vi "OCV Histogram.vi"() -> ()   [LabVIEW 2019]
uses:
  OCVResults.ctl
  <vilib>/Analysis/baseanly.llb/Mean (DBL).vi
  <vilib>/Analysis/NI_AALBase.lvlib
  <vilib>/gmath/NI_Gmath.lvlib
panel:
  in  "Shorted at Pogo Pins":T1={"V ch0 Array"=[-4.644502656163076e-06, -5.008064093958253e-06, -5.142051723342297e-06, -4.750005660824572e-06, -4.652031142446432e-06, -5.209066755986695e-06, -5.091916834616591e-06, -4.630381027105227e-06, -5.21237404687769e-06, -5.620858205189846e-06, -5.343550677180362e-06, -6.185703766713982e-06, -5.671664561333461e-06, -5.927670894878171e-06, -5.546613668877613e-06, -6.364344983296889e-06, -6.520646681657183e-06, -6.284866762207373e-06, -6.533935582056949e-06, -6.4689426016067465e-06, -6.593996925988968e-06, -6.285432522003292e-06, -6.408103781833046e-06, -7.058105327323116e-06, -6.870211305723346e-06, -6.925936314908492e-06, -7.1087845232367935e-06, -6.979415887004172e-06, -7.113203152470592e-06, -6.8704523945523955e-06, -7.009159603790376e-06, -7.342517581426176e-06, -7.669098159443e-06, -7.489677328220809e-06, -7.132610877720342e-06, -7.304233870876275e-06, -7.66832379992834e-06, -7.715296105424593e-06, -7.986434127352774e-06, -7.898970931824006e-06], "V ch1 Array"=[4.7742232260821556e-06, 4.920022255268294e-06, 4.483256762256209e-06, 4.404065475875136e-06, 4.4716932731421325e-06, 4.548985062890386e-06, 4.522408472375412e-06, 4.095669599355476e-06, 3.999328189678911e-06, 3.6813476852782265e-06, 3.872005693197737e-06, 3.758508170269238e-06, 3.70571748427637e-06, 3.4759885510773306e-06, 2.9599721164895703e-06, 2.7610141257932504e-06, 2.8118433858193503e-06, 2.7104175464413036e-06, 2.565833035431353e-06, 2.185911565670746e-06, 2.685980675088301e-06, 2.6488195890091604e-06, 2.076266606944392e-06, 2.2698362478026414e-06, 1.5578322743180792e-06, 1.5376996626048395e-06, 1.150473677761539e-06, 1.8236979091692574e-06, 1.510963150770623e-06, 1.4855862808683257e-06, 1.4125163986427117e-06, 1.0735262618997076e-06, 9.45720576216451e-07, 4.7672136505507866e-07, 9.053063870402968e-07, 6.054055041162458e-07, 4.721349816794846e-07, 5.456028909058344e-07, 3.3431927350417376e-07, -1.5058882941009345e-07], "V ch2 Array"=[1.4134743604832099e-05, 1.3658244443019425e-05, 1.3479236357815262e-05, 1.367186906530213e-05, 1.2455842044663626e-05, 1.3434705047662445e-05, 1.3432391541088278e-05, 1.2888375409531819e-05, 1.2977936688443777e-05, 1.2674364164577651e-05, 1.2242971027474285e-05, 1.2123410935032508e-05, 1.1563631234108194e-05, 1.1923757910255661e-05, 1.1189143138664649e-05, 1.0898907804721548e-05, 1.0581785706128752e-05, 1.056110705533516e-05, 1.0471726258982195e-05, 1.0112137397062614e-05, 1.0207095545974621e-05, 1.0393895961777352e-05, 9.905291985333096e-06, 9.553343876750542e-06, 8.558186802328226e-06, 8.88351705449872e-06, 7.898230501439385e-06, 8.415417566964899e-06, 8.559435016019298e-06, 7.776376116877038e-06, 7.927651129172682e-06, 7.5739375202025605e-06, 7.10207278100178e-06, 6.5660504928688425e-06, 7.061106613490489e-06, 6.858259813662034e-06, 6.848030448614549e-06, 6.09752727757034e-06, 6.274361642967703e-06, 6.342704065028583e-06], "V ch3 Array"=[6.213352398330788e-06, 6.334228296782694e-06, 6.080028793939261e-06, 6.247654310029223e-06, 5.7595966055769634e-06, 5.814589345926128e-06, 5.6246681289139826e-06, 5.644165962745353e-06, 5.6293504739542166e-06, 5.352467720756411e-06, 5.130425551487793e-06, 5.1973648252728e-06, 5.044212335842026e-06, 4.8718454017924225e-06, 4.157122967118985e-06, 4.067943871712763e-06, 4.140736203520263e-06, 3.6541795943306613e-06, 4.0305384502788036e-06, 4.0890937751910164e-06, 3.7562699778786177e-06, 3.6969730552191906e-06, 3.508773289214503e-06, 3.4081260252248884e-06, 2.849755744581444e-06, 2.9121416252580047e-06, 2.743264262706753e-06, 2.425566322314393e-06, 2.3612672502798895e-06, 2.3528107196359356e-06, 2.284734780010105e-06, 2.0191213502578e-06, 1.7636078290436924e-06, 2.2789345039783042e-06, 1.9002135193771114e-06, 1.991552898527243e-06, 1.8062353830205049e-06, 1.382185125377262e-06, 1.10266330045512e-06, 1.2689722392645079e-06], "V ch4 Array"=[7.418128083831304e-06, 6.737017232964174e-06, 7.37695117366581e-06, 7.383316471897266e-06, 6.9171589884302516e-06, 6.824032641156624e-06, 7.123351361466038e-06, 6.907639604422655e-06, 6.77516452363689e-06, 6.995953660130747e-06, 6.47180172880639e-06, 6.431905767977081e-06, 6.870003361647515e-06, 6.6674721347179e-06, 6.65655896542764e-06, 5.8891322446061865e-06, 6.26132019363544e-06, 5.653457993699113e-06, 5.979464421600547e-06, 6.0940365547306505e-06, 5.726374609261477e-06, 5.609776313356894e-06, 5.925170773010799e-06, 5.980594209927675e-06, 5.615200324832046e-06, 5.423645487579083e-06, 4.863795777172752e-06, 5.24223894551309e-06, 4.7771857502833714e-06, 5.20649511681379e-06, 4.976881377243475e-06, 4.382659410631824e-06, 4.409179837473124e-06, 5.0132045585108375e-06, 4.846028587433284e-06, 5.007743407280303e-06, 5.115217349204208e-06, 4.756883872606744e-06, 4.378539859901796e-06, 4.191624122691694e-06], "Elapsed Time (ms)"=41178, "DMM Fault Array"=[FALSE, FALSE, FALSE, FALSE, FALSE, FALSE, FALSE, FALSE, FALSE, FALSE, FALSE, FALSE, FALSE, FALSE, FALSE, FALSE, FALSE, FALSE, FALSE, FALSE, FALSE, FALSE, FALSE, FALSE, FALSE, FALSE, FALSE, FALSE, FALSE, FALSE, FALSE, FALSE, FALSE, FALSE, FALSE, FALSE, FALSE, FALSE, FALSE, FALSE, FALSE, FALSE, FALSE, FALSE, FALSE, FALSE, FALSE, FALSE, FALSE, FALSE, FALSE, FALSE, FALSE, FALSE, FALSE, FALSE, FALSE, FALSE, FALSE, FALSE, FALSE, FALSE, FALSE, FALSE, FALSE, FALSE, FALSE, FALSE, FALSE, FALSE, FALSE, FALSE, FALSE, FALSE, FALSE, FALSE, FALSE, FALSE, FALSE, FALSE, FALSE, FALSE, FALSE, FALSE, FALSE, FALSE, FALSE, FALSE, FALSE, FALSE, FALSE, FALSE, FALSE, FALSE, FALSE, FALSE, FALSE, FALSE, FALSE, FALSE, FALSE, FALSE, FALSE, FALSE, FALSE, FALSE, FALSE, FALSE, FALSE, FALSE, FALSE, FALSE, FALSE, FALSE, FALSE, FALSE, FALSE, FALSE, FALSE, FALSE, FALSE, FALSE, FALSE, FALSE, FALSE, FALSE, FALSE, FALSE, FALSE, FALSE, FALSE, FALSE, FALSE, FALSE, FALSE, FALSE, FALSE, FALSE, FALSE, FALSE, FALSE, FALSE, FALSE, FALSE, FALSE, FALSE, FALSE, FALSE, FALSE, FALSE, FALSE, FALSE, FALSE, FALSE, FALSE, FALSE, FALSE, FALSE, FALSE, FALSE, FALSE, FALSE, FALSE, FALSE, FALSE, FALSE, FALSE, FALSE, FALSE, FALSE, FALSE, FALSE, FALSE, FALSE, FALSE, FALSE, FALSE, FALSE, FALSE, FALSE, FALSE, FALSE, FALSE, FALSE, FALSE, FALSE, FALSE, FALSE, FALSE, FALSE, FALSE, FALSE, FALSE, FALSE, FALSE, FALSE, FALSE, FALSE, FALSE, FALSE]}
  out "mean values of channels":dbl[](array[numeric])=[3.4860065278089722, 3.48375553663424, 3.4808778023254034, 3.484652928409848, 3.4829310355717924] format="%#_7p"
  in  "Aperture 200ms":T1={"V ch0 Array"=[3.486008136472735, 3.48600857919526, 3.486008593885945, 3.486008866783261, 3.48600839296004, 3.4860084310246897, 3.4860079537562934, 3.486008185287128, 3.486007910716225, 3.486008248243466, 3.486008226064088, 3.4860074977647457, 3.4860073987599094, 3.4860073866023904, 3.486006180409399, 3.486007074730973, 3.486007704925445, 3.4860074052013497, 3.4860071909298775, 3.486007294352636, 3.4860070893197057, 3.486006585724478, 3.4860062950330795, 3.486005770351729, 3.486006470228577, 3.486006294219978, 3.486006261625677, 3.486005971624855, 3.4860053268849924, 3.486005293813216, 3.4860057372410087, 3.4860055538519807, 3.486004986165897, 3.486005215637336, 3.4860050104743285, 3.4860054747400397, 3.486005352423458, 3.486005243822349, 3.4860053543618483, 3.4860050193699643], "V ch1 Array"=[3.483761574282832, 3.4837611271000504, 3.483761800210414, 3.4837619249854033, 3.4837611548851593, 3.483760899396786, 3.483761030316352, 3.4837614126693177, 3.483761111670994, 3.483761223907113, 3.4837605553855715, 3.483760811426642, 3.483760756142808, 3.483760849802524, 3.48376001298478, 3.4837605620529932, 3.483760624523579, 3.4837598644530314, 3.4837598021350367, 3.483759678841745, 3.483759236759767, 3.483759830079179, 3.4837586449222844, 3.4837592160716793, 3.4837591729619493, 3.4837584791863603, 3.4837585600417578, 3.483758759299516, 3.483758443826462, 3.4837582905594657, 3.483758319275863, 3.4837578525324924, 3.483757492097309, 3.483758508843088, 3.483758252435504, 3.4837583290172742, 3.4837582653066366, 3.4837580432257322, 3.4837579872411233, 3.4837572297984027], "V ch2 Array"=[3.480887331125, 3.4808873642804303, 3.4808872284950985, 3.4808870880116816, 3.480886718645805, 3.480886569722079, 3.480886668360947, 3.480887124574677, 3.4808868556225554, 3.4808863352702843, 3.480886374563708, 3.4808863195405926, 3.480885492039432, 3.480885499125927, 3.4808853435833824, 3.480885304255472, 3.4808854048927067, 3.480885548024527, 3.4808846074916104, 3.480884933260716, 3.480884045102653, 3.4808848759996445, 3.4808834564381117, 3.480884092168976, 3.4808840639635292, 3.4808839119975015, 3.480884117918731, 3.4808838222854104, 3.4808837132230104, 3.480882970525138, 3.4808832280724213, 3.480882799469968, 3.4808825004595314, 3.4808829485765864, 3.4808825054329224, 3.480882618811386, 3.480882555023867, 3.4808814816354365, 3.4808821449010603, 3.480881613246818], "V ch3 Array"=[3.4846494420325933, 3.4846499531928408, 3.484649881478528, 3.484649477663704, 3.484649028003101, 3.4846491662272117, 3.484648764064297, 3.484649038455092, 3.4846488791274033, 3.4846493802112795, 3.484648500366631, 3.4846488541657643, 3.484647926389134, 3.484647926012707, 3.4846477409134877, 3.4846480348803968, 3.4846481902030244, 3.4846476677611595, 3.484647180925758, 3.4846471596264443, 3.48464679726762, 3.484647693286154, 3.484646021250072, 3.4846464856341806, 3.48464646608778, 3.4846465629811068, 3.4846461202335623, 3.484646282076445, 3.484645610465135, 3.4846448549897504, 3.484645234223203, 3.484644743913154, 3.4846449104812334, 3.484645286668683, 3.4846446745957183, 3.4846443026433325, 3.484644591867837, 3.484643852000993, 3.4846443663887183, 3.4846437781492234], "V ch4 Array"=[3.4829266330342312, 3.482927618195819, 3.4829267375359523, 3.482926673878544, 3.482926361108386, 3.482926051177458, 3.4829261918098164, 3.482926643011778, 3.4829263973622697, 3.4829267486003386, 3.482926239361367, 3.482926009047662, 3.4829255763196625, 3.4829252649644946, 3.482926010999456, 3.4829256561545856, 3.482925616603878, 3.482925430299697, 3.482925384824906, 3.482925111093104, 3.4829243773568472, 3.4829245855818627, 3.4829236684214164, 3.4829243150207865, 3.48292388842584, 3.482924459144899, 3.4829244509598785, 3.4829235506462766, 3.4829238640017737, 3.4829231152951126, 3.4829231533373095, 3.4829234989073856, 3.482923429513632, 3.482923569887466, 3.4829233778303514, 3.48292294148491, 3.4829225870708402, 3.482922885194255, 3.48292277091393, 3.482922191039904], "Elapsed Time (ms)"=41179, "DMM Fault Array"=[FALSE, FALSE, FALSE, FALSE, FALSE, FALSE, FALSE, FALSE, FALSE, FALSE, FALSE, FALSE, FALSE, FALSE, FALSE, FALSE, FALSE, FALSE, FALSE, FALSE, FALSE, FALSE, FALSE, FALSE, FALSE, FALSE, FALSE, FALSE, FALSE, FALSE, FALSE, FALSE, FALSE, FALSE, FALSE, FALSE, FALSE, FALSE, FALSE, FALSE, FALSE, FALSE, FALSE, FALSE, FALSE, FALSE, FALSE, FALSE, FALSE, FALSE, FALSE, FALSE, FALSE, FALSE, FALSE, FALSE, FALSE, FALSE, FALSE, FALSE, FALSE, FALSE, FALSE, FALSE, FALSE, FALSE, FALSE, FALSE, FALSE, FALSE, FALSE, FALSE, FALSE, FALSE, FALSE, FALSE, FALSE, FALSE, FALSE, FALSE, FALSE, FALSE, FALSE, FALSE, FALSE, FALSE, FALSE, FALSE, FALSE, FALSE, FALSE, FALSE, FALSE, FALSE, FALSE, FALSE, FALSE, FALSE, FALSE, FALSE, FALSE, FALSE, FALSE, FALSE, FALSE, FALSE, FALSE, FALSE, FALSE, FALSE, FALSE, FALSE, FALSE, FALSE, FALSE, FALSE, FALSE, FALSE, FALSE, FALSE, FALSE, FALSE, FALSE, FALSE, FALSE, FALSE, FALSE, FALSE, FALSE, FALSE, FALSE, FALSE, FALSE, FALSE, FALSE, FALSE, FALSE, FALSE, FALSE, FALSE, FALSE, FALSE, FALSE, FALSE, FALSE, FALSE, FALSE, FALSE, FALSE, FALSE, FALSE, FALSE, FALSE, FALSE, FALSE, FALSE, FALSE, FALSE, FALSE, FALSE, FALSE, FALSE, FALSE, FALSE, FALSE, FALSE, FALSE, FALSE, FALSE, FALSE, FALSE, FALSE, FALSE, FALSE, FALSE, FALSE, FALSE, FALSE, FALSE, FALSE, FALSE, FALSE, FALSE, FALSE, FALSE, FALSE, FALSE, FALSE, FALSE, FALSE, FALSE, FALSE, FALSE, FALSE, FALSE, FALSE, FALSE, FALSE, FALSE, FALSE]}
  in  "Aperture 100ms":T1={"V ch0 Array"=[3.486009342585924, 3.4860105791739295, 3.486009931293131, 3.4860104287389, 3.4860092107388985, 3.486010141865981, 3.4860099876219555, 3.4860099847912083, 3.4860105815524287, 3.4860097585412158, 3.486009884787763, 3.4860103699490104, 3.4860101319846923, 3.4860100232587925, 3.4860097575418165, 3.4860098656116585, 3.4860099281665464, 3.4860101703729627, 3.4860095171681698, 3.486009274858784, 3.486008835388769, 3.4860101964727264, 3.4860099208454622, 3.486009396754712, 3.486009765859615, 3.4860100085572148, 3.486009761006136, 3.4860093507563175, 3.486010114650017, 3.486010095359039, 3.486009239422696, 3.486009747196399, 3.4860095662543613, 3.486009897920948, 3.4860090987744554, 3.4860091306648, 3.4860088161589653, 3.4860087248708242, 3.486008795417955, 3.4860089917588786], "V ch1 Array"=[3.4837624269768077, 3.48376228114691, 3.4837624931669393, 3.483761690503522, 3.483762155112424, 3.4837623742938635, 3.483762530621196, 3.4837625073929708, 3.4837629531752388, 3.4837628311532667, 3.4837623445473884, 3.4837624893774435, 3.4837624783754726, 3.4837629314944056, 3.4837620420976028, 3.4837623355175706, 3.4837620224590617, 3.4837628211868528, 3.4837625542351085, 3.4837617678834287, 3.4837613820224265, 3.4837629202530915, 3.483762550398443, 3.483762098662157, 3.483762194447779, 3.483762525958178, 3.4837624272950842, 3.4837620308215613, 3.4837620769856987, 3.483762428084855, 3.4837614921239366, 3.4837618093626643, 3.483761940909492, 3.483762461616833, 3.483761691185677, 3.4837617745493117, 3.483761713223301, 3.4837616040814634, 3.4837614420599667, 3.48376097030803], "V ch2 Array"=[3.4808881795721174, 3.4808883313716246, 3.480888898340563, 3.480888295742587, 3.480888608550977, 3.4808887791773486, 3.4808884610442696, 3.480888665380878, 3.4808884002018616, 3.4808887742205608, 3.480887630055783, 3.4808880675947815, 3.4808884701480265, 3.4808883902919048, 3.4808881624179406, 3.4808878492628614, 3.480888261000973, 3.4808883629946665, 3.4808881818180226, 3.4808876522799888, 3.480887461292375, 3.480888607451478, 3.480887839077484, 3.4808872769077657, 3.4808874503677765, 3.4808875084242965, 3.4808873046245945, 3.4808874834171952, 3.480886785383865, 3.480886872329251, 3.4808875891233906, 3.480887116764498, 3.480886791395762, 3.480887286883312, 3.4808869352248015, 3.4808867541286497, 3.4808863857441597, 3.480886392902343, 3.480886055482132, 3.480885490000428], "V ch3 Array"=[3.484651699388893, 3.484651545846978, 3.4846512315009237, 3.4846512380454784, 3.4846516053658094, 3.4846518730555442, 3.484651375621465, 3.4846524671533308, 3.484651872127177, 3.484651836357751, 3.4846512940631733, 3.484651339393445, 3.484651943755441, 3.484651992458054, 3.484650533966351, 3.484650906778825, 3.4846514868400833, 3.4846515569158076, 3.4846513629276004, 3.4846508460654917, 3.484650626430101, 3.4846512615447227, 3.4846506421425434, 3.484651362249249, 3.4846503023743085, 3.4846507344492568, 3.484650635547321, 3.4846504986168716, 3.484650507900654, 3.484650249934964, 3.484650813855195, 3.484649807825047, 3.484649765228285, 3.48465038699218, 3.484649863980596, 3.484649023843705, 3.4846489818429665, 3.484649383129509, 3.484649201493699, 3.4846489918759493], "V ch4 Array"=[3.482927735803894, 3.482927340280007, 3.482927450118009, 3.482927667247653, 3.482927828334824, 3.4829274360243563, 3.482928060851357, 3.4829282380460005, 3.482927707338127, 3.482927638010684, 3.48292776532699, 3.4829276207246203, 3.482928248308542, 3.4829279098062047, 3.4829276721732416, 3.4829277669695853, 3.4829282785856024, 3.4829278902480967, 3.482927734684043, 3.482927119973658, 3.482927618691812, 3.482927625774665, 3.4829269275383856, 3.4829274148488474, 3.4829274061226, 3.4829269572792154, 3.4829273071837483, 3.482928083458411, 3.482928213245571, 3.4829277993020136, 3.4829274353081385, 3.4829265960951377, 3.4829273450195637, 3.4829272886160374, 3.4829269443181414, 3.482926203898658, 3.4829261490935757, 3.4829262414280016, 3.4829262680441184, 3.482925750053477], "Elapsed Time (ms)"=21179, "DMM Fault Array"=[FALSE, FALSE, FALSE, FALSE, FALSE, FALSE, FALSE, FALSE, FALSE, FALSE, FALSE, FALSE, FALSE, FALSE, FALSE, FALSE, FALSE, FALSE, FALSE, FALSE, FALSE, FALSE, FALSE, FALSE, FALSE, FALSE, FALSE, FALSE, FALSE, FALSE, FALSE, FALSE, FALSE, FALSE, FALSE, FALSE, FALSE, FALSE, FALSE, FALSE, FALSE, FALSE, FALSE, FALSE, FALSE, FALSE, FALSE, FALSE, FALSE, FALSE, FALSE, FALSE, FALSE, FALSE, FALSE, FALSE, FALSE, FALSE, FALSE, FALSE, FALSE, FALSE, FALSE, FALSE, FALSE, FALSE, FALSE, FALSE, FALSE, FALSE, FALSE, FALSE, FALSE, FALSE, FALSE, FALSE, FALSE, FALSE, FALSE, FALSE, FALSE, FALSE, FALSE, FALSE, FALSE, FALSE, FALSE, FALSE, FALSE, FALSE, FALSE, FALSE, FALSE, FALSE, FALSE, FALSE, FALSE, FALSE, FALSE, FALSE, FALSE, FALSE, FALSE, FALSE, FALSE, FALSE, FALSE, FALSE, FALSE, FALSE, FALSE, FALSE, FALSE, FALSE, FALSE, FALSE, FALSE, FALSE, FALSE, FALSE, FALSE, FALSE, FALSE, FALSE, FALSE, FALSE, FALSE, FALSE, FALSE, FALSE, FALSE, FALSE, FALSE, FALSE, FALSE, FALSE, FALSE, FALSE, FALSE, FALSE, FALSE, FALSE, FALSE, FALSE, FALSE, FALSE, FALSE, FALSE, FALSE, FALSE, FALSE, FALSE, FALSE, FALSE, FALSE, FALSE, FALSE, FALSE, FALSE, FALSE, FALSE, FALSE, FALSE, FALSE, FALSE, FALSE, FALSE, FALSE, FALSE, FALSE, FALSE, FALSE, FALSE, FALSE, FALSE, FALSE, FALSE, FALSE, FALSE, FALSE, FALSE, FALSE, FALSE, FALSE, FALSE, FALSE, FALSE, FALSE, FALSE, FALSE, FALSE, FALSE, FALSE, FALSE, FALSE, FALSE, FALSE, FALSE, FALSE, FALSE]}
  in  "Aperture 83.333ms":T1={"V ch0 Array"=[3.486011308516991, 3.486012239712371, 3.4860117488002986, 3.4860117846643788, 3.4860112460509, 3.4860122062360275, 3.486011836169301, 3.486012369801971, 3.4860122187882556, 3.486012566602132, 3.4860122523310664, 3.4860122171529238, 3.4860121108134354, 3.4860123157743494, 3.4860122873127923, 3.4860124760718674, 3.486012337141422, 3.4860116684592, 3.4860121407169955, 3.4860121021406, 3.4860123592450254, 3.486012151457661, 3.486012121814877, 3.486012067279236, 3.4860123631776054, 3.4860121056043045, 3.4860114488809137, 3.486011754799218, 3.4860106856009794, 3.4860112875473717, 3.486011703795938, 3.4860120408526933, 3.4860107437568857, 3.48601088290282, 3.4860113654835745, 3.486011077482956, 3.486011198731769, 3.4860110498434973, 3.4860110418920347, 3.4860114222959866], "V ch1 Array"=[3.48376144514735, 3.483762834467521, 3.4837631670672375, 3.4837623545770247, 3.483762107595157, 3.4837626511367517, 3.483762686272187, 3.483763061857131, 3.483762799687585, 3.483763256237141, 3.4837627216036235, 3.4837630898972405, 3.4837625437622455, 3.483763470688663, 3.483763332566706, 3.4837632413297466, 3.4837632297716534, 3.483763046847993, 3.483762554574395, 3.4837626769665397, 3.483763593758579, 3.4837636694535936, 3.4837630032740696, 3.4837637224866063, 3.4837629548968807, 3.4837628958155715, 3.4837626640538226, 3.4837626122337526, 3.483762711500467, 3.483762055280072, 3.483762819116541, 3.4837627515538023, 3.483761992186221, 3.4837623338946315, 3.4837620187762153, 3.483761909221837, 3.483762264846845, 3.4837623892072913, 3.4837624615777685, 3.483762348335557], "V ch2 Array"=[3.480888708513571, 3.4808899222268774, 3.4808891805476914, 3.480890012447383, 3.4808892224486154, 3.4808893541433874, 3.4808892866436536, 3.480890020112137, 3.4808897263400347, 3.480889783586903, 3.480889935849121, 3.4808896507279634, 3.480889351773294, 3.480890064216353, 3.4808901385444586, 3.4808896580000983, 3.480889498764669, 3.4808898293598274, 3.4808895506765243, 3.480889693145708, 3.480889162389052, 3.4808896927476467, 3.4808892966308354, 3.4808899571134586, 3.480889465662438, 3.4808889111399703, 3.480888409068941, 3.480888525715946, 3.4808890429173713, 3.4808889264302345, 3.4808885737492994, 3.480888487697757, 3.480888024775162, 3.4808879516614852, 3.4808876036613943, 3.4808880185797495, 3.4808879533956265, 3.4808879726788993, 3.4808881120797213, 3.480887678005953], "V ch3 Array"=[3.4846535014569993, 3.4846541760292356, 3.484653522898726, 3.4846537234499997, 3.484654274868219, 3.4846541533184623, 3.4846538790205623, 3.484653703267222, 3.4846537737054746, 3.484654159822945, 3.484654165902905, 3.484654192635321, 3.484654175425727, 3.4846535327376635, 3.484653580198149, 3.484654506816064, 3.4846534264712856, 3.484653785252615, 3.484653990393246, 3.4846533736484147, 3.4846532689913223, 3.484653468831708, 3.4846538432365963, 3.4846537804540145, 3.4846535567722334, 3.4846528159762866, 3.4846519071808677, 3.4846523265662555, 3.484652590816005, 3.484651964351458, 3.4846524738855367, 3.4846523590459872, 3.484652375375891, 3.484652087227577, 3.484651774761584, 3.484651925046, 3.4846519185425966, 3.4846519450610187, 3.4846520067304745, 3.4846515142009595], "V ch4 Array"=[3.4829264000035693, 3.4829270474083764, 3.4829273700349654, 3.48292728310475, 3.482927554955438, 3.4829280842549744, 3.482928116817796, 3.4829269335611985, 3.4829284615526284, 3.4829276929963067, 3.482928105095857, 3.4829276890211416, 3.482927228135068, 3.482927749550447, 3.4829278369724954, 3.4829277993952084, 3.482928003490174, 3.4829275404308224, 3.48292756348699, 3.482927639736477, 3.482926867361093, 3.4829272666686393, 3.482927349826675, 3.482927777135856, 3.482926506905905, 3.482926708523178, 3.482927039514058, 3.482926967607869, 3.482926263410761, 3.482926437644337, 3.4829274705024393, 3.482926618936467, 3.482926341189578, 3.48292661596785, 3.4829265616882217, 3.4829265081437066, 3.4829261104994833, 3.4829263487877005, 3.4829268727396743, 3.4829262442480986], "Elapsed Time (ms)"=17840, "DMM Fault Array"=[FALSE, FALSE, FALSE, FALSE, FALSE, FALSE, FALSE, FALSE, FALSE, FALSE, FALSE, FALSE, FALSE, FALSE, FALSE, FALSE, FALSE, FALSE, FALSE, FALSE, FALSE, FALSE, FALSE, FALSE, FALSE, FALSE, FALSE, FALSE, FALSE, FALSE, FALSE, FALSE, FALSE, FALSE, FALSE, FALSE, FALSE, FALSE, FALSE, FALSE, FALSE, FALSE, FALSE, FALSE, FALSE, FALSE, FALSE, FALSE, FALSE, FALSE, FALSE, FALSE, FALSE, FALSE, FALSE, FALSE, FALSE, FALSE, FALSE, FALSE, FALSE, FALSE, FALSE, FALSE, FALSE, FALSE, FALSE, FALSE, FALSE, FALSE, FALSE, FALSE, FALSE, FALSE, FALSE, FALSE, FALSE, FALSE, FALSE, FALSE, FALSE, FALSE, FALSE, FALSE, FALSE, FALSE, FALSE, FALSE, FALSE, FALSE, FALSE, FALSE, FALSE, FALSE, FALSE, FALSE, FALSE, FALSE, FALSE, FALSE, FALSE, FALSE, FALSE, FALSE, FALSE, FALSE, FALSE, FALSE, FALSE, FALSE, FALSE, FALSE, FALSE, FALSE, FALSE, FALSE, FALSE, FALSE, FALSE, FALSE, FALSE, FALSE, FALSE, FALSE, FALSE, FALSE, FALSE, FALSE, FALSE, FALSE, FALSE, FALSE, FALSE, FALSE, FALSE, FALSE, FALSE, FALSE, FALSE, FALSE, FALSE, FALSE, FALSE, FALSE, FALSE, FALSE, FALSE, FALSE, FALSE, FALSE, FALSE, FALSE, FALSE, FALSE, FALSE, FALSE, FALSE, FALSE, FALSE, FALSE, FALSE, FALSE, FALSE, FALSE, FALSE, FALSE, FALSE, FALSE, FALSE, FALSE, FALSE, FALSE, FALSE, FALSE, FALSE, FALSE, FALSE, FALSE, FALSE, FALSE, FALSE, FALSE, FALSE, FALSE, FALSE, FALSE, FALSE, FALSE, FALSE, FALSE, FALSE, FALSE, FALSE, FALSE, FALSE, FALSE, FALSE, FALSE, FALSE, FALSE]}
  in  "Aperture 66.666ms":T1={"V ch0 Array"=[3.4860087998577005, 3.4860095881357007, 3.4860101243172754, 3.4860101144901403, 3.486009888487567, 3.4860095771678257, 3.486009669258281, 3.4860094591080513, 3.4860103646585396, 3.4860097369646823, 3.4860096987264826, 3.486009571351648, 3.4860098771934167, 3.4860097835806916, 3.486009561905741, 3.486010032506046, 3.4860089841340414, 3.4860092949017023, 3.4860102057709037, 3.4860095439580023, 3.486010152423206, 3.4860106769541708, 3.486010233961671, 3.4860094919269367, 3.4860097824232867, 3.4860095692285054, 3.486009586955168, 3.486009895817203, 3.486010327033842, 3.486009759381219, 3.4860098017300087, 3.4860101603499363, 3.4860098840038014, 3.4860099658133556, 3.486009908145774, 3.486009609018681, 3.4860096586646816, 3.486009804783706, 3.4860093085592134, 3.486009478902439], "V ch1 Array"=[3.483760919705666, 3.483761869245746, 3.483761959360454, 3.4837610510443393, 3.4837611770683603, 3.4837613541505483, 3.483761535168446, 3.4837615945078113, 3.483762097514668, 3.4837613706486406, 3.483761473980138, 3.483761884265854, 3.4837617247467976, 3.4837617012079223, 3.483760834123308, 3.483761090501802, 3.48376059513931, 3.4837613052709315, 3.483762005734639, 3.4837610896972415, 3.4837617908589684, 3.4837615663936834, 3.483761747238985, 3.4837616692609985, 3.483761646197544, 3.483761294896974, 3.4837604944369978, 3.483761837306543, 3.4837615877681896, 3.4837618075102377, 3.4837615882889503, 3.483761703673241, 3.483761248077784, 3.483761700151896, 3.4837612726209124, 3.483760588068086, 3.4837613416844158, 3.4837609694613487, 3.483760924435762, 3.4837608925182137], "V ch2 Array"=[3.4808863773772543, 3.480886669418454, 3.4808873886157263, 3.480886413588629, 3.4808873618899736, 3.4808873437807266, 3.480886755177445, 3.4808869453382223, 3.480887464165299, 3.480886900782393, 3.4808870436569843, 3.4808874679648922, 3.4808870994368517, 3.4808865690442543, 3.480886784455878, 3.4808868210363446, 3.4808859487488313, 3.4808868680223597, 3.480886776757931, 3.480886801707026, 3.480887196454042, 3.480887405892581, 3.4808876132499544, 3.480886555301745, 3.480886529704909, 3.480886739877629, 3.4808865320412967, 3.480887301554799, 3.480886582542384, 3.4808868800235953, 3.480886739982213, 3.4808867859782278, 3.4808864774264436, 3.480886305721363, 3.4808861528966646, 3.4808867325743194, 3.4808864343840265, 3.480886312203627, 3.480886584938389, 3.48088646297481], "V ch3 Array"=[3.484650807229959, 3.484651774283296, 3.4846519516933347, 3.4846516319475054, 3.484652063235418, 3.484652071854816, 3.4846516202986617, 3.4846517014537373, 3.4846523194092835, 3.4846521211999524, 3.484651702162199, 3.4846519295670677, 3.4846517340825005, 3.4846513680635502, 3.4846512057138934, 3.4846515287948328, 3.4846519286333084, 3.484651188287481, 3.484651349773111, 3.484651995793708, 3.4846520150992184, 3.4846522758834984, 3.4846518137849802, 3.484651297913903, 3.4846510243965803, 3.484651358305008, 3.484651452402426, 3.4846524632395934, 3.484651705527652, 3.484651694168373, 3.4846516821692313, 3.4846512991773837, 3.4846514629860112, 3.484650672181916, 3.4846509088214157, 3.484650732648704, 3.484650894748678, 3.4846505911642187, 3.484651294143712, 3.4846510357548985], "V ch4 Array"=[3.4829272996810947, 3.4829272782624443, 3.4829275139775517, 3.4829269004471395, 3.4829275408550995, 3.4829277689113125, 3.4829271335226237, 3.4829276730931262, 3.4829268209667936, 3.482927367613094, 3.482927607066623, 3.4829268691426827, 3.4829268903447055, 3.4829273896280197, 3.482927105499838, 3.4829262932216025, 3.482927081371735, 3.4829266027300334, 3.48292673298539, 3.482927489707926, 3.48292727137664, 3.4829276427095914, 3.4829278822666185, 3.482926515712328, 3.482926621734275, 3.482927051972468, 3.48292694912251, 3.4829277226679234, 3.482927064940792, 3.4829270499583376, 3.482927283643157, 3.482927446903043, 3.482927333199049, 3.482926437014769, 3.48292713227865, 3.482926646534637, 3.482926836756891, 3.482926598365688, 3.482926850846762, 3.4829269468668755], "Elapsed Time (ms)"=14513, "DMM Fault Array"=[FALSE, FALSE, FALSE, FALSE, FALSE, FALSE, FALSE, FALSE, FALSE, FALSE, FALSE, FALSE, FALSE, FALSE, FALSE, FALSE, FALSE, FALSE, FALSE, FALSE, FALSE, FALSE, FALSE, FALSE, FALSE, FALSE, FALSE, FALSE, FALSE, FALSE, FALSE, FALSE, FALSE, FALSE, FALSE, FALSE, FALSE, FALSE, FALSE, FALSE, FALSE, FALSE, FALSE, FALSE, FALSE, FALSE, FALSE, FALSE, FALSE, FALSE, FALSE, FALSE, FALSE, FALSE, FALSE, FALSE, FALSE, FALSE, FALSE, FALSE, FALSE, FALSE, FALSE, FALSE, FALSE, FALSE, FALSE, FALSE, FALSE, FALSE, FALSE, FALSE, FALSE, FALSE, FALSE, FALSE, FALSE, FALSE, FALSE, FALSE, FALSE, FALSE, FALSE, FALSE, FALSE, FALSE, FALSE, FALSE, FALSE, FALSE, FALSE, FALSE, FALSE, FALSE, FALSE, FALSE, FALSE, FALSE, FALSE, FALSE, FALSE, FALSE, FALSE, FALSE, FALSE, FALSE, FALSE, FALSE, FALSE, FALSE, FALSE, FALSE, FALSE, FALSE, FALSE, FALSE, FALSE, FALSE, FALSE, FALSE, FALSE, FALSE, FALSE, FALSE, FALSE, FALSE, FALSE, FALSE, FALSE, FALSE, FALSE, FALSE, FALSE, FALSE, FALSE, FALSE, FALSE, FALSE, FALSE, FALSE, FALSE, FALSE, FALSE, FALSE, FALSE, FALSE, FALSE, FALSE, FALSE, FALSE, FALSE, FALSE, FALSE, FALSE, FALSE, FALSE, FALSE, FALSE, FALSE, FALSE, FALSE, FALSE, FALSE, FALSE, FALSE, FALSE, FALSE, FALSE, FALSE, FALSE, FALSE, FALSE, FALSE, FALSE, FALSE, FALSE, FALSE, FALSE, FALSE, FALSE, FALSE, FALSE, FALSE, FALSE, FALSE, FALSE, FALSE, FALSE, FALSE, FALSE, FALSE, FALSE, FALSE, FALSE, FALSE, FALSE, FALSE, FALSE, FALSE, FALSE]}
  in  "Aperture 50ms":T1={"V ch0 Array"=[3.4860100287152176, 3.4860105188849553, 3.4860106708159453, 3.4860094634778664, 3.4860099118737806, 3.486010523724517, 3.4860099052381313, 3.4860102303967886, 3.4860101301121498, 3.486010292651811, 3.486010199771339, 3.4860106853911876, 3.4860109895623905, 3.4860107133588483, 3.486010447394096, 3.4860106566610725, 3.486010997892429, 3.4860101234952126, 3.48600996479348, 3.486010103181317, 3.4860105876357554, 3.48601023084213, 3.486009867094396, 3.4860098108988984, 3.4860092398388813, 3.486009725324624, 3.4860096603576003, 3.486008896488685, 3.4860092704556815, 3.4860095697732945, 3.486008558194004, 3.4860089610080696, 3.486008673120214, 3.4860087699924494, 3.4860092785317387, 3.486009367161149, 3.486009226546915, 3.4860096822694366, 3.4860096977392105, 3.4860099169280505], "V ch1 Array"=[3.4837622547034077, 3.4837615815666485, 3.483762529014476, 3.4837621681655278, 3.483762188707288, 3.4837618633463263, 3.483763227201614, 3.4837621427685534, 3.483762683392615, 3.4837623289394593, 3.4837627534166558, 3.48376346772014, 3.4837636251775055, 3.483762457405858, 3.4837634794729304, 3.483762977481437, 3.4837629345679324, 3.4837631030207246, 3.4837629456461694, 3.4837628484726055, 3.483761997597191, 3.4837625049740137, 3.483762216727805, 3.4837620043126956, 3.48376213159136, 3.483762096545265, 3.4837617435558927, 3.4837615058818554, 3.4837615885265003, 3.4837616255565362, 3.4837616788541252, 3.4837613812367385, 3.4837609512517314, 3.4837611696355744, 3.483761983589698, 3.483761966858258, 3.4837613659045283, 3.4837618682766567, 3.483761915919694, 3.4837619313026145], "V ch2 Array"=[3.4808869609246615, 3.480887261550433, 3.4808881245642356, 3.480887435501162, 3.4808866862045176, 3.480887868244338, 3.4808878821670226, 3.4808874703312456, 3.4808879690318433, 3.480888364513961, 3.480888033583846, 3.4808881142078136, 3.4808884304361305, 3.4808877278394137, 3.480888662188628, 3.480888094184551, 3.480887905268431, 3.480888371276923, 3.4808875432440796, 3.4808870941774988, 3.480887088434577, 3.480886791269301, 3.4808872805992475, 3.48088653865037, 3.4808866413425985, 3.4808865319189217, 3.48088656482604, 3.480886159814531, 3.4808860148618375, 3.480886538568749, 3.4808863033367845, 3.4808863711956852, 3.480886349091009, 3.480886181851329, 3.480886257965578, 3.4808862479847065, 3.4808864937119854, 3.480885765574369, 3.4808864743103074, 3.480887148388446], "V ch3 Array"=[3.4846509510160764, 3.4846510772479133, 3.4846514563068767, 3.4846511988461897, 3.4846505946638815, 3.4846512096738143, 3.4846517813774347, 3.4846511706468046, 3.4846511446643524, 3.4846514268988478, 3.4846516574479858, 3.4846511067785237, 3.4846520394102742, 3.484651878669274, 3.4846515793422235, 3.484651904943696, 3.4846511309148287, 3.4846514308431367, 3.4846516282787454, 3.484650023138923, 3.484651163887891, 3.484650193990817, 3.4846513598563225, 3.4846500346856906, 3.4846499656426575, 3.4846498234359946, 3.4846503795494663, 3.4846493936957663, 3.4846497630741227, 3.4846502843060607, 3.484649841027079, 3.4846493597248243, 3.484649892599996, 3.4846501778195464, 3.484650363201697, 3.484650494803555, 3.4846496243922878, 3.48464972852744, 3.4846500119053396, 3.484650533730012], "V ch4 Array"=[3.4829269850420745, 3.482927590238761, 3.482926653853842, 3.4829272143652914, 3.482927514085087, 3.482926705112038, 3.4829271862570357, 3.482926691178922, 3.482927613190633, 3.4829280914145424, 3.4829273547258395, 3.4829278085809356, 3.4829273448330196, 3.4829267716041663, 3.4829274831376797, 3.4829276839601047, 3.48292753499368, 3.48292751625691, 3.482926970155153, 3.482927468403634, 3.482927606619747, 3.482926889628744, 3.482927135801245, 3.4829262477892695, 3.4829270214994756, 3.4829260292107223, 3.4829260559211996, 3.482926067329125, 3.482926268835784, 3.482926248827354, 3.4829258919295123, 3.4829255437612, 3.482925544229328, 3.482925454846341, 3.4829265604884223, 3.4829256645431097, 3.482925571973606, 3.4829265171301365, 3.4829258623487998, 3.4829263404476105], "Elapsed Time (ms)"=11163, "DMM Fault Array"=[FALSE, FALSE, FALSE, FALSE, FALSE, FALSE, FALSE, FALSE, FALSE, FALSE, FALSE, FALSE, FALSE, FALSE, FALSE, FALSE, FALSE, FALSE, FALSE, FALSE, FALSE, FALSE, FALSE, FALSE, FALSE, FALSE, FALSE, FALSE, FALSE, FALSE, FALSE, FALSE, FALSE, FALSE, FALSE, FALSE, FALSE, FALSE, FALSE, FALSE, FALSE, FALSE, FALSE, FALSE, FALSE, FALSE, FALSE, FALSE, FALSE, FALSE, FALSE, FALSE, FALSE, FALSE, FALSE, FALSE, FALSE, FALSE, FALSE, FALSE, FALSE, FALSE, FALSE, FALSE, FALSE, FALSE, FALSE, FALSE, FALSE, FALSE, FALSE, FALSE, FALSE, FALSE, FALSE, FALSE, FALSE, FALSE, FALSE, FALSE, FALSE, FALSE, FALSE, FALSE, FALSE, FALSE, FALSE, FALSE, FALSE, FALSE, FALSE, FALSE, FALSE, FALSE, FALSE, FALSE, FALSE, FALSE, FALSE, FALSE, FALSE, FALSE, FALSE, FALSE, FALSE, FALSE, FALSE, FALSE, FALSE, FALSE, FALSE, FALSE, FALSE, FALSE, FALSE, FALSE, FALSE, FALSE, FALSE, FALSE, FALSE, FALSE, FALSE, FALSE, FALSE, FALSE, FALSE, FALSE, FALSE, FALSE, FALSE, FALSE, FALSE, FALSE, FALSE, FALSE, FALSE, FALSE, FALSE, FALSE, FALSE, FALSE, FALSE, FALSE, FALSE, FALSE, FALSE, FALSE, FALSE, FALSE, FALSE, FALSE, FALSE, FALSE, FALSE, FALSE, FALSE, FALSE, FALSE, FALSE, FALSE, FALSE, FALSE, FALSE, FALSE, FALSE, FALSE, FALSE, FALSE, FALSE, FALSE, FALSE, FALSE, FALSE, FALSE, FALSE, FALSE, FALSE, FALSE, FALSE, FALSE, FALSE, FALSE, FALSE, FALSE, FALSE, FALSE, FALSE, FALSE, FALSE, FALSE, FALSE, FALSE, FALSE, FALSE, FALSE, FALSE, FALSE, FALSE, FALSE]}
  in  "Aperture 33.333ms":T1={"V ch0 Array"=[3.486008824721795, 3.4860102954706935, 3.4860102805490536, 3.4860104842509556, 3.486010439216268, 3.4860097506123746, 3.4860094118729426, 3.4860095021603867, 3.486009978947523, 3.4860098527233068, 3.4860104496716957, 3.4860103895692003, 3.486010367848577, 3.48601062969307, 3.486010983039664, 3.486010601867436, 3.4860103471495156, 3.486010350156111, 3.4860109559511416, 3.486010623693404, 3.4860099601058097, 3.486009678156399, 3.4860099554361725, 3.486010964829207, 3.486011070196151, 3.4860102335975793, 3.486009795616894, 3.486009791478988, 3.4860103649925387, 3.4860105454214105, 3.4860103593221274, 3.4860097590006656, 3.4860102750790807, 3.4860098695304615, 3.486009689969913, 3.486009765170063, 3.486010633744698, 3.4860097948422704, 3.4860108150506823, 3.4860103815675147], "V ch1 Array"=[3.4837603258260885, 3.4837617209091727, 3.4837607054841624, 3.4837608669525584, 3.483761387972808, 3.4837605276830113, 3.4837601763707005, 3.48376106793701, 3.4837612224269385, 3.483760134780626, 3.483760344510397, 3.483761034988426, 3.4837603752016095, 3.483761524629875, 3.483760448725977, 3.483760844175594, 3.4837608280042622, 3.483760771288343, 3.4837608177320876, 3.4837609751564123, 3.483760553479603, 3.4837607902877195, 3.483760468508287, 3.483761524541938, 3.48376177388621, 3.48376108279076, 3.483760791124656, 3.483760627368547, 3.4837612265244586, 3.48376107354724, 3.4837609476556985, 3.4837599947813955, 3.483760991018429, 3.4837606629534483, 3.483760104440811, 3.4837599418879694, 3.4837600619779963, 3.4837603916271487, 3.483760031432464, 3.48376071776108], "V ch2 Array"=[3.480885648500254, 3.480886623417331, 3.4808860498699996, 3.480886186354761, 3.480886518964582, 3.4808866154115994, 3.480886086431394, 3.480886212991607, 3.4808867856130297, 3.4808867840557216, 3.480886067282028, 3.4808864524076855, 3.480886483395374, 3.4808864287799537, 3.480886062446561, 3.4808860458316664, 3.480885981048711, 3.4808860556304055, 3.4808858829924376, 3.4808857395291954, 3.4808856791543095, 3.4808857345631496, 3.4808866935924505, 3.480886065264016, 3.4808868453322033, 3.4808859301600323, 3.4808863097002334, 3.4808859380467223, 3.4808865198463215, 3.480886518985954, 3.4808865525070756, 3.4808859541073085, 3.480886566420257, 3.4808855235340044, 3.4808857303615053, 3.4808852225286726, 3.480885004070249, 3.4808850374398297, 3.4808848368048024, 3.4808854169617702], "V ch3 Array"=[3.484650789693503, 3.484651250197442, 3.4846508071905666, 3.4846511027113487, 3.484650758221049, 3.48465152442972, 3.484651246169689, 3.4846516080847234, 3.484652411100253, 3.4846515404879854, 3.484651498259433, 3.4846515257284842, 3.4846516276101442, 3.484652211977694, 3.484651634146663, 3.4846509892179687, 3.4846508115968184, 3.484651645337553, 3.484651146860917, 3.484650633655282, 3.484650893968318, 3.4846509741598095, 3.484651317065715, 3.4846513969926707, 3.4846517059426008, 3.4846516345650502, 3.4846517748899344, 3.4846521467734766, 3.484651960231268, 3.4846518031150056, 3.484652440777864, 3.4846514939552717, 3.484651610968441, 3.4846515970746927, 3.4846518484096274, 3.484651222128941, 3.4846515349380804, 3.4846520362195825, 3.484651247241264, 3.48465109769376], "V ch4 Array"=[3.4829252966293796, 3.482926195359479, 3.4829258655676596, 3.482925582683675, 3.4829250655263944, 3.4829253970040717, 3.482925409412919, 3.482926195188618, 3.4829262089248263, 3.4829257568466443, 3.4829258700497645, 3.4829268007989627, 3.48292644572667, 3.4829264671455125, 3.482926297934609, 3.4829256212157547, 3.482926069008827, 3.482926043793742, 3.482926060870626, 3.4829265015533704, 3.4829256411231784, 3.4829254188328145, 3.4829254139004733, 3.482925931192824, 3.4829257033362926, 3.4829257286206605, 3.4829253685503145, 3.4829260452900406, 3.4829249228985693, 3.4829253371595823, 3.4829258729745307, 3.482925361591034, 3.482925810317688, 3.4829262633234457, 3.4829253729081646, 3.4829252234308714, 3.4829258557394693, 3.482926538721085, 3.4829257679098857, 3.4829255344908825], "Elapsed Time (ms)"=7822, "DMM Fault Array"=[FALSE, FALSE, FALSE, FALSE, FALSE, FALSE, FALSE, FALSE, FALSE, FALSE, FALSE, FALSE, FALSE, FALSE, FALSE, FALSE, FALSE, FALSE, FALSE, FALSE, FALSE, FALSE, FALSE, FALSE, FALSE, FALSE, FALSE, FALSE, FALSE, FALSE, FALSE, FALSE, FALSE, FALSE, FALSE, FALSE, FALSE, FALSE, FALSE, FALSE, FALSE, FALSE, FALSE, FALSE, FALSE, FALSE, FALSE, FALSE, FALSE, FALSE, FALSE, FALSE, FALSE, FALSE, FALSE, FALSE, FALSE, FALSE, FALSE, FALSE, FALSE, FALSE, FALSE, FALSE, FALSE, FALSE, FALSE, FALSE, FALSE, FALSE, FALSE, FALSE, FALSE, FALSE, FALSE, FALSE, FALSE, FALSE, FALSE, FALSE, FALSE, FALSE, FALSE, FALSE, FALSE, FALSE, FALSE, FALSE, FALSE, FALSE, FALSE, FALSE, FALSE, FALSE, FALSE, FALSE, FALSE, FALSE, FALSE, FALSE, FALSE, FALSE, FALSE, FALSE, FALSE, FALSE, FALSE, FALSE, FALSE, FALSE, FALSE, FALSE, FALSE, FALSE, FALSE, FALSE, FALSE, FALSE, FALSE, FALSE, FALSE, FALSE, FALSE, FALSE, FALSE, FALSE, FALSE, FALSE, FALSE, FALSE, FALSE, FALSE, FALSE, FALSE, FALSE, FALSE, FALSE, FALSE, FALSE, FALSE, FALSE, FALSE, FALSE, FALSE, FALSE, FALSE, FALSE, FALSE, FALSE, FALSE, FALSE, FALSE, FALSE, FALSE, FALSE, FALSE, FALSE, FALSE, FALSE, FALSE, FALSE, FALSE, FALSE, FALSE, FALSE, FALSE, FALSE, FALSE, FALSE, FALSE, FALSE, FALSE, FALSE, FALSE, FALSE, FALSE, FALSE, FALSE, FALSE, FALSE, FALSE, FALSE, FALSE, FALSE, FALSE, FALSE, FALSE, FALSE, FALSE, FALSE, FALSE, FALSE, FALSE, FALSE, FALSE, FALSE, FALSE, FALSE, FALSE, FALSE]}
  in  "Aperture 16.666ms":T1={"V ch0 Array"=[3.4860106218117752, 3.4860125747320114, 3.486011373017407, 3.4860074813288304, 3.4860080959449626, 3.4860120329456583, 3.4860130219387244, 3.486007954916858, 3.4860067792110594, 3.4860113773209656, 3.4860127432118784, 3.486008719451372, 3.4860064281386305, 3.486008992393793, 3.4860129146099945, 3.48601273638565, 3.48600760017669, 3.4860070802179717, 3.4860120640227152, 3.4860144314593176, 3.486009648377591, 3.486007608016022, 3.486009646858304, 3.4860125988705915, 3.486012350233539, 3.4860086408469058, 3.48600756225683, 3.4860114364225327, 3.48601430984272, 3.4860090888836335, 3.4860063599458035, 3.4860106301157905, 3.486012144427349, 3.486009721504358, 3.486006061150122, 3.4860079521781175, 3.4860118730588345, 3.486012828523596, 3.4860081145774116, 3.486006062719392], "V ch1 Array"=[3.4837572471223295, 3.483757173205013, 3.483763245006702, 3.483763566091828, 3.483758701422186, 3.483756940584071, 3.4837616350451697, 3.4837643800870848, 3.4837607070428103, 3.4837569071227494, 3.4837588110996403, 3.483762889029664, 3.483762886098842, 3.483757206448899, 3.483756569055416, 3.4837632691137976, 3.48376453629407, 3.483760313725405, 3.4837577450281194, 3.4837599003883057, 3.483763400370334, 3.4837633765649145, 3.483758358248541, 3.4837579119832935, 3.483762583085892, 3.4837662628589823, 3.48376030574225, 3.4837568474654512, 3.4837606936853573, 3.4837637714222947, 3.4837623995655065, 3.4837575926050035, 3.4837573739655747, 3.4837628087948493, 3.4837640996712147, 3.4837587236991214, 3.483757432878568, 3.4837611496565457, 3.483764679287454, 3.483760788583478], "V ch2 Array"=[3.480889295801355, 3.480885405967352, 3.480883103587753, 3.4808861853162933, 3.480889636723398, 3.4808877622427996, 3.4808828455747283, 3.4808837607122864, 3.4808875761460993, 3.4808890897982567, 3.480884293499084, 3.480882896344634, 3.48088575268319, 3.480888211980551, 3.480885953061376, 3.480882439466244, 3.4808850033310623, 3.4808889984810008, 3.480889229246013, 3.480884428944085, 3.4808833247266415, 3.4808881324947234, 3.4808900218630057, 3.480886752517301, 3.480882497552943, 3.480885035053463, 3.4808886113227286, 3.480888249289288, 3.480884364816636, 3.480883942219394, 3.4808869102772246, 3.4808888605102197, 3.4808855282883826, 3.4808827363829375, 3.4808842370797137, 3.4808889874630897, 3.4808868354203115, 3.4808828856744656, 3.4808833516671593, 3.4808880221072713], "V ch3 Array"=[3.4846498683134937, 3.4846540517586524, 3.4846533579758905, 3.484649348521892, 3.4846488237740196, 3.48465348887773, 3.484654428552599, 3.4846506852445756, 3.4846490931629432, 3.48465226751673, 3.484655249966371, 3.4846532897459794, 3.484647982607527, 3.4846496398230853, 3.484653777491491, 3.484654872463534, 3.4846502524443213, 3.484648839981512, 3.4846519052738714, 3.484655738517453, 3.4846536804848585, 3.4846486238562777, 3.484649407461698, 3.4846546290911595, 3.4846555902243606, 3.4846504340612436, 3.4846490668589443, 3.484652137605248, 3.484654994881213, 3.4846525468959832, 3.4846476539425235, 3.484650524775551, 3.4846544525194356, 3.4846536414823888, 3.484648991511996, 3.4846486085059856, 3.4846537264533883, 3.4846548854106665, 3.4846518206925428, 3.484648720522117], "V ch4 Array"=[3.4829242161394802, 3.4829235930569276, 3.4829290119597993, 3.4829311505983847, 3.4829264747276643, 3.482923378103817, 3.482926458676701, 3.4829306103800017, 3.482929520759486, 3.4829253536711953, 3.482924570946773, 3.48292978430578, 3.482930903802149, 3.4829253961042674, 3.482923495431282, 3.4829278682615064, 3.4829322799399347, 3.4829299704154253, 3.482925063486103, 3.482925508122742, 3.482930334557988, 3.4829328545768123, 3.4829260354459994, 3.482924346373963, 3.4829288783530368, 3.4829316514879434, 3.4829281804150996, 3.4829255733819515, 3.482925744296375, 3.482930554164376, 3.482931549479858, 3.482925789079616, 3.4829248117468725, 3.482928882987789, 3.4829313489318756, 3.4829278542815727, 3.4829234062126173, 3.482926978290302, 3.482930813804889, 3.4829298408289735], "Elapsed Time (ms)"=4463, "DMM Fault Array"=[FALSE, FALSE, FALSE, FALSE, FALSE, FALSE, FALSE, FALSE, FALSE, FALSE, FALSE, FALSE, FALSE, FALSE, FALSE, FALSE, FALSE, FALSE, FALSE, FALSE, FALSE, FALSE, FALSE, FALSE, FALSE, FALSE, FALSE, FALSE, FALSE, FALSE, FALSE, FALSE, FALSE, FALSE, FALSE, FALSE, FALSE, FALSE, FALSE, FALSE, FALSE, FALSE, FALSE, FALSE, FALSE, FALSE, FALSE, FALSE, FALSE, FALSE, FALSE, FALSE, FALSE, FALSE, FALSE, FALSE, FALSE, FALSE, FALSE, FALSE, FALSE, FALSE, FALSE, FALSE, FALSE, FALSE, FALSE, FALSE, FALSE, FALSE, FALSE, FALSE, FALSE, FALSE, FALSE, FALSE, FALSE, FALSE, FALSE, FALSE, FALSE, FALSE, FALSE, FALSE, FALSE, FALSE, FALSE, FALSE, FALSE, FALSE, FALSE, FALSE, FALSE, FALSE, FALSE, FALSE, FALSE, FALSE, FALSE, FALSE, FALSE, FALSE, FALSE, FALSE, FALSE, FALSE, FALSE, FALSE, FALSE, FALSE, FALSE, FALSE, FALSE, FALSE, FALSE, FALSE, FALSE, FALSE, FALSE, FALSE, FALSE, FALSE, FALSE, FALSE, FALSE, FALSE, FALSE, FALSE, FALSE, FALSE, FALSE, FALSE, FALSE, FALSE, FALSE, FALSE, FALSE, FALSE, FALSE, FALSE, FALSE, FALSE, FALSE, FALSE, FALSE, FALSE, FALSE, FALSE, FALSE, FALSE, FALSE, FALSE, FALSE, FALSE, FALSE, FALSE, FALSE, FALSE, FALSE, FALSE, FALSE, FALSE, FALSE, FALSE, FALSE, FALSE, FALSE, FALSE, FALSE, FALSE, FALSE, FALSE, FALSE, FALSE, FALSE, FALSE, FALSE, FALSE, FALSE, FALSE, FALSE, FALSE, FALSE, FALSE, FALSE, FALSE, FALSE, FALSE, FALSE, FALSE, FALSE, FALSE, FALSE, FALSE, FALSE, FALSE, FALSE, FALSE, FALSE, FALSE]}
  in  "6.5 Digit - 200 Measurements - AZonce ADCCaloff":T1={"V ch0 Array"=[3.4860098572964087, 3.4860104437518005, 3.486010456404461, 3.486010775112258, 3.486010669658029, 3.486010697824209, 3.48601076821764, 3.4860109024978785, 3.4860105839623796, 3.48601107999324, 3.486011260392315, 3.486011414117023, 3.4860114633894055, 3.486010963574942, 3.486010943068894, 3.486010713437261, 3.4860109640727606, 3.486011128681875, 3.4860110229037042, 3.4860104429334635, 3.486010049619942, 3.4860103470551533, 3.4860104905028013, 3.4860104803474425, 3.486010076866105, 3.486009207313286, 3.486009737129387, 3.486009534066967, 3.486009375585875, 3.4860092157987195, 3.4860092199489254, 3.486009330559762, 3.486009603328705, 3.4860093121555953, 3.4860089369931635, 3.4860085568165835, 3.4860090556814547, 3.486009432584104, 3.4860095823908988, 3.48600923715036], "V ch1 Array"=[3.4837615500127295, 3.483761898826035, 3.483761801799038, 3.483762023604336, 3.483762053187564, 3.4837623500720176, 3.483762029396489, 3.483761409975747, 3.4837618572057756, 3.4837626194485556, 3.4837619927427426, 3.4837618124527365, 3.4837622878855568, 3.483762203929324, 3.4837617780951806, 3.483761859757461, 3.483761606256813, 3.483762076556962, 3.483761648189091, 3.4837612120773027, 3.4837611681271516, 3.4837609580649884, 3.4837615790977816, 3.4837613060484456, 3.483760967863254, 3.483760763745215, 3.4837610911242924, 3.4837607360413068, 3.483760034334831, 3.483760532344684, 3.483760318914922, 3.483760773950178, 3.48376033151435, 3.483760197521679, 3.48375982481605, 3.483759598193658, 3.4837602852311758, 3.483760478415968, 3.4837598419250586, 3.4837605871137076], "V ch2 Array"=[3.4808864317794455, 3.4808866413015855, 3.4808871957024548, 3.4808868406462685, 3.480887150890017, 3.480887093702329, 3.4808875476070114, 3.4808872955271437, 3.4808867638864514, 3.4808875108380306, 3.480886834120402, 3.4808866984025513, 3.480886820401143, 3.4808868430788866, 3.480886661081383, 3.480886303400147, 3.4808870776669596, 3.4808874213629686, 3.4808862272956453, 3.4808860649904845, 3.480885184493842, 3.4808859491270367, 3.4808863654593734, 3.480885674343702, 3.480885437958592, 3.480885416461691, 3.48088501735329, 3.4808852472560443, 3.480885510499157, 3.4808844557355716, 3.4808850296750355, 3.480885193986261, 3.480884607069066, 3.4808847063467705, 3.4808844451871543, 3.4808844981371845, 3.4808843334436514, 3.4808840733934656, 3.480884422252361, 3.4808843489686265], "V ch3 Array"=[3.4846547176104354, 3.4846547806134547, 3.4846551638171213, 3.484654926205374, 3.484655200551438, 3.484655612253781, 3.484655203277421, 3.4846550695286336, 3.484655440924673, 3.4846558498979574, 3.484655660677341, 3.4846552311832193, 3.4846556374780255, 3.4846555240949995, 3.484654517708969, 3.4846545327991363, 3.484655309052153, 3.4846552548597662, 3.484654683617297, 3.484654359463488, 3.4846538297885643, 3.4846542065916375, 3.484654052400227, 3.4846538576297688, 3.484653806845705, 3.4846530708306216, 3.4846533440661407, 3.484653436239468, 3.484652797294846, 3.4846527862591876, 3.4846523446087443, 3.4846523100499276, 3.4846526565847635, 3.484652217680419, 3.484652571744781, 3.4846521046081746, 3.4846522971054856, 3.484652012840219, 3.484652243432274, 3.4846514986805994], "V ch4 Array"=[3.4829309758956466, 3.482930861822449, 3.4829306633476613, 3.482931276968647, 3.4829312196277944, 3.4829316251140705, 3.482930749565874, 3.4829306616480937, 3.4829313013345478, 3.4829311489627344, 3.4829316606980587, 3.482931253116037, 3.4829310389117247, 3.482931047321298, 3.4829307864132044, 3.482930497691867, 3.482931275207294, 3.482930723578534, 3.4829309387530833, 3.4829298553611747, 3.48293057323363, 3.4829306831999998, 3.482930868330645, 3.4829306893264547, 3.482930070735135, 3.4829299732915278, 3.4829297579015353, 3.482929695441859, 3.4829294951090435, 3.482928683774882, 3.4829295512155496, 3.482929731132313, 3.482929003012163, 3.482929566280308, 3.482929094696708, 3.4829294516638014, 3.482929719528548, 3.4829291804884024, 3.4829292602114394, 3.482929085134734], "Elapsed Time (ms)"=21181, "DMM Fault Array"=[FALSE, FALSE, FALSE, FALSE, FALSE, FALSE, FALSE, FALSE, FALSE, FALSE, FALSE, FALSE, FALSE, FALSE, FALSE, FALSE, FALSE, FALSE, FALSE, FALSE, FALSE, FALSE, FALSE, FALSE, FALSE, FALSE, FALSE, FALSE, FALSE, FALSE, FALSE, FALSE, FALSE, FALSE, FALSE, FALSE, FALSE, FALSE, FALSE, FALSE, FALSE, FALSE, FALSE, FALSE, FALSE, FALSE, FALSE, FALSE, FALSE, FALSE, FALSE, FALSE, FALSE, FALSE, FALSE, FALSE, FALSE, FALSE, FALSE, FALSE, FALSE, FALSE, FALSE, FALSE, FALSE, FALSE, FALSE, FALSE, FALSE, FALSE, FALSE, FALSE, FALSE, FALSE, FALSE, FALSE, FALSE, FALSE, FALSE, FALSE, FALSE, FALSE, FALSE, FALSE, FALSE, FALSE, FALSE, FALSE, FALSE, FALSE, FALSE, FALSE, FALSE, FALSE, FALSE, FALSE, FALSE, FALSE, FALSE, FALSE, FALSE, FALSE, FALSE, FALSE, FALSE, FALSE, FALSE, FALSE, FALSE, FALSE, FALSE, FALSE, FALSE, FALSE, FALSE, FALSE, FALSE, FALSE, FALSE, FALSE, FALSE, FALSE, FALSE, FALSE, FALSE, FALSE, FALSE, FALSE, FALSE, FALSE, FALSE, FALSE, FALSE, FALSE, FALSE, FALSE, FALSE, FALSE, FALSE, FALSE, FALSE, FALSE, FALSE, FALSE, FALSE, FALSE, FALSE, FALSE, FALSE, FALSE, FALSE, FALSE, FALSE, FALSE, FALSE, FALSE, FALSE, FALSE, FALSE, FALSE, FALSE, FALSE, FALSE, FALSE, FALSE, FALSE, FALSE, FALSE, FALSE, FALSE, FALSE, FALSE, FALSE, FALSE, FALSE, FALSE, FALSE, FALSE, FALSE, FALSE, FALSE, FALSE, FALSE, FALSE, FALSE, FALSE, FALSE, FALSE, FALSE, FALSE, FALSE, FALSE, FALSE, FALSE, FALSE, FALSE, FALSE, FALSE, FALSE, FALSE]}
  out "range":dbl=5.505011136541782e-06 format="%.3p"
  out "std dev":dbl=1.5335351881596951e-06 format="%.3p"
  out "mean":dbl=3.4836447661500514 format="%.6p"
  in  "3.5 Digit - 200 Measurements":T1={"V ch0 Array"=[3.4860103075998685, 3.486012058575334, 3.485992797845221, 3.4859980507716157, 3.4860278173545165, 3.4860173115017288, 3.4859962997961507, 3.4860085566244043, 3.4859998017470812, 3.4860120585753336, 3.4859962997961516, 3.4859945488206865, 3.486020813452657, 3.485987544918827, 3.48600330369801, 3.486005054673476, 3.486008556624404, 3.4859770390660403, 3.48601030759987, 3.4859875449188267, 3.4860190624771925, 3.4860330702809104, 3.485994548820687, 3.4860120585753345, 3.486020813452658, 3.4860033036980105, 3.4860068056489384, 3.4860400741827697, 3.4860190624771925, 3.486012058575333, 3.4860313193054475, 3.4860260663790523, 3.486019062477193, 3.486012058575334, 3.48597353711511, 3.48599629979615, 3.48603657223184, 3.486019062477193, 3.4859805410169686, 3.486019062477193], "V ch1 Array"=[3.4837427943730486, 3.483741043397583, 3.483772560955948, 3.4837690590050188, 3.4837585531522306, 3.4837743119314126, 3.4837760629068786, 3.4837655570540895, 3.483755051201301, 3.483751549250371, 3.483734039495724, 3.483763806078625, 3.4837445453485127, 3.4837848177842012, 3.48375855315223, 3.4837533002258367, 3.4837533002258363, 3.48378831973513, 3.4837147787656124, 3.483730537544794, 3.4837515492503712, 3.4837462963239765, 3.483741043397583, 3.4837620551031585, 3.4837708099804834, 3.4837883197351296, 3.4837497982749075, 3.483756802176765, 3.483737541446654, 3.4837357904711883, 3.4837603041276948, 3.483763806078625, 3.483756802176765, 3.4837900707105955, 3.483779564857807, 3.483746296323978, 3.4837848177842012, 3.4837603041276943, 3.4837620551031594, 3.483763806078625], "V ch2 Array"=[3.4808589377826413, 3.4808834514391482, 3.480907965095654, 3.4808887043655425, 3.48090621412019, 3.480890455341008, 3.480900961193795, 3.480920221923907, 3.4808764475372893, 3.480899210218331, 3.4808624397335715, 3.4809044631447255, 3.4808974592428643, 3.4808781985127544, 3.480886953390079, 3.4808904553410076, 3.4808939572919364, 3.480883451439148, 3.4808992102183307, 3.480895708267401, 3.4808992102183303, 3.4808746965618247, 3.4808904553410063, 3.4808711946108954, 3.4808554358317116, 3.480858937782642, 3.480885202414613, 3.4808764475372893, 3.4808746965618242, 3.4808746965618242, 3.480888704365543, 3.480902712169261, 3.4808904553410067, 3.480897459242866, 3.4808694436354304, 3.4808887043655417, 3.4808781985127544, 3.4809079650956547, 3.4808799494882185, 3.480881700463685], "V ch3 Array"=[3.4846515506392426, 3.484646297712847, 3.4846830681976053, 3.4846410447864535, 3.4846603055165644, 3.484662056492029, 3.4846550525901705, 3.484646297712847, 3.48465505259017, 3.4846515506392404, 3.4846287879582003, 3.4846585545410997, 3.484669060393889, 3.484672562344818, 3.4846462977128465, 3.4846743133202827, 3.484674313320282, 3.4846585545410993, 3.484651550639241, 3.4846620564920294, 3.4846585545410997, 3.484635791860059, 3.484632289909128, 3.4846445467373814, 3.4846603055165644, 3.4846813172221416, 3.484681317222142, 3.484642795761917, 3.4846865701485346, 3.484627036982735, 3.4846445467373823, 3.4846550525901705, 3.4846515506392413, 3.4846217840563405, 3.4846270369827343, 3.4846480486883125, 3.4846568035656356, 3.484665558442958, 3.4846620564920294, 3.4846375428355243], "V ch4 Array"=[3.482909330051838, 3.482928590781949, 3.482919835904626, 3.4829110810273023, 3.4828918202971906, 3.482921586880091, 3.482949602487526, 3.48292508883102, 3.482911081027303, 3.482930341757415, 3.4829180849291608, 3.4829425985856677, 3.482912832002767, 3.48292508883102, 3.482933843708344, 3.4829373456592725, 3.4829128320027665, 3.482954855413921, 3.4829145829782315, 3.4829531044384554, 3.482947851512062, 3.482951353462991, 3.4829390966347393, 3.482937345659274, 3.482918084929162, 3.482949602487527, 3.4829461005365965, 3.482923337855556, 3.4829671122421737, 3.4829320927328786, 3.4829215868800913, 3.482953104438456, 3.482916333953697, 3.482935594683808, 3.482953104438456, 3.482919835904626, 3.482923337855555, 3.4829408476102026, 3.4829408476102026, 3.482911081027302], "Elapsed Time (ms)"=1317, "DMM Fault Array"=[FALSE, FALSE, FALSE, FALSE, FALSE, FALSE, FALSE, FALSE, FALSE, FALSE, FALSE, FALSE, FALSE, FALSE, FALSE, FALSE, FALSE, FALSE, FALSE, FALSE, FALSE, FALSE, FALSE, FALSE, FALSE, FALSE, FALSE, FALSE, FALSE, FALSE, FALSE, FALSE, FALSE, FALSE, FALSE, FALSE, FALSE, FALSE, FALSE, FALSE, FALSE, FALSE, FALSE, FALSE, FALSE, FALSE, FALSE, FALSE, FALSE, FALSE, FALSE, FALSE, FALSE, FALSE, FALSE, FALSE, FALSE, FALSE, FALSE, FALSE, FALSE, FALSE, FALSE, FALSE, FALSE, FALSE, FALSE, FALSE, FALSE, FALSE, FALSE, FALSE, FALSE, FALSE, FALSE, FALSE, FALSE, FALSE, FALSE, FALSE, FALSE, FALSE, FALSE, FALSE, FALSE, FALSE, FALSE, FALSE, FALSE, FALSE, FALSE, FALSE, FALSE, FALSE, FALSE, FALSE, FALSE, FALSE, FALSE, FALSE, FALSE, FALSE, FALSE, FALSE, FALSE, FALSE, FALSE, FALSE, FALSE, FALSE, FALSE, FALSE, FALSE, FALSE, FALSE, FALSE, FALSE, FALSE, FALSE, FALSE, FALSE, FALSE, FALSE, FALSE, FALSE, FALSE, FALSE, FALSE, FALSE, FALSE, FALSE, FALSE, FALSE, FALSE, FALSE, FALSE, FALSE, FALSE, FALSE, FALSE, FALSE, FALSE, FALSE, FALSE, FALSE, FALSE, FALSE, FALSE, FALSE, FALSE, FALSE, FALSE, FALSE, FALSE, FALSE, FALSE, FALSE, FALSE, FALSE, FALSE, FALSE, FALSE, FALSE, FALSE, FALSE, FALSE, FALSE, FALSE, FALSE, FALSE, FALSE, FALSE, FALSE, FALSE, FALSE, FALSE, FALSE, FALSE, FALSE, FALSE, FALSE, FALSE, FALSE, FALSE, FALSE, FALSE, FALSE, FALSE, FALSE, FALSE, FALSE, FALSE, FALSE, FALSE, FALSE, FALSE, FALSE, FALSE, FALSE, FALSE]}
  in  "4.5 Digit - 200 Measurements":T1={"V ch0 Array"=[3.486059334912881, 3.48606633881474, 3.4860558329619513, 3.486068089790204, 3.4860540819864867, 3.4860295683299802, 3.4860803466184582, 3.4860523310110216, 3.4860593349128806, 3.486031319305447, 3.4860243154035864, 3.4860505800355583, 3.4860225644281213, 3.486029568329981, 3.486024315403587, 3.486012058575334, 3.4860383232073033, 3.486020813452657, 3.4860330702809104, 3.486073342716599, 3.4860278173545165, 3.486048829060093, 3.4860365722318405, 3.4860383232073042, 3.48603657223184, 3.4860540819864876, 3.486055832961952, 3.4860540819864863, 3.4860610858883465, 3.4860628368638107, 3.4860680897902045, 3.486075093692064, 3.486061085888346, 3.486031319305446, 3.486045327109163, 3.4860278173545156, 3.4860365722318396, 3.4860313193054457, 3.4860260663790505, 3.486075093692063], "V ch1 Array"=[3.4837918216860597, 3.483777813882342, 3.483812833391636, 3.4837865687596654, 3.4838233392444238, 3.4837760629068777, 3.483805829489778, 3.483812833391636, 3.4837953236369894, 3.483776062906877, 3.48382158826896, 3.483807580465242, 3.483807580465243, 3.4838040785143125, 3.48378831973513, 3.483797074612453, 3.483767308029555, 3.4837813158332716, 3.483786568759666, 3.4837970746124545, 3.483798825587919, 3.483783066808736, 3.483783066808737, 3.4837603041276948, 3.4837760629068772, 3.483798825587918, 3.4837725609559484, 3.4837743119314126, 3.483779564857807, 3.4838461019254656, 3.483797074612454, 3.4837865687596654, 3.4838005765633833, 3.4837865687596663, 3.483784817784201, 3.4838093314407077, 3.4838215882689596, 3.483800576563384, 3.4837848177842003, 3.4837865687596663], "V ch2 Array"=[3.480937731678555, 3.4809499885068074, 3.4808939572919355, 3.480946486555878, 3.4809149689975123, 3.4809307277766948, 3.4809202219239075, 3.4809377316785537, 3.4808904553410067, 3.4809324787521607, 3.480914968997513, 3.4808992102183303, 3.4809132180220486, 3.480914968997513, 3.4809114670465835, 3.480930727776696, 3.4809219728993717, 3.4809394826540196, 3.4809079650956534, 3.480907965095654, 3.4809552414332017, 3.480923723874837, 3.4809289768012297, 3.4809184709484424, 3.480914968997513, 3.4809237238748367, 3.480902712169259, 3.4809254748503022, 3.480925474850301, 3.4809307277766957, 3.4809429846049498, 3.4808852024146124, 3.4809079650956543, 3.4809237238748363, 3.4809377316785546, 3.480937731678556, 3.480909716071119, 3.480927225825766, 3.480923723874837, 3.4809009611937958], "V ch3 Array"=[3.4846638074674945, 3.484688321124, 3.4846865701485363, 3.4846883211239996, 3.484719838682365, 3.4846830681976058, 3.4846900720994647, 3.4847180877069, 3.4846743133202827, 3.484726842584224, 3.484691823074929, 3.4847040799031825, 3.484691823074929, 3.4847075818541122, 3.4846603055165644, 3.4846743133202813, 3.4847040799031825, 3.484695325025859, 3.484677815271213, 3.484702328927718, 3.4847058308786476, 3.4847110838050424, 3.484695325025859, 3.484665558442958, 3.484684819173071, 3.484667309418423, 3.484705830878647, 3.4846708113693534, 3.484702328927718, 3.4846795662466765, 3.484681317222142, 3.4846638074674936, 3.484674313320282, 3.484672562344817, 3.4846620564920285, 3.4847163367314358, 3.48468481917307, 3.4847233406332934, 3.4846900720994647, 3.4846935740503944], "V ch4 Array"=[3.482954855413919, 3.482940847610203, 3.4829373456592734, 3.482947851512061, 3.4829618593157785, 3.482944349561132, 3.4829303417574136, 3.4829566063893855, 3.482972365168568, 3.4829583573648497, 3.482979369070426, 3.4829741161440326, 3.4829706141931025, 3.482970614193102, 3.4829968788250745, 3.482982871021357, 3.4829741161440326, 3.4829793690704265, 3.482939096634738, 3.4829513534629912, 3.4830091356533264, 3.482981120045891, 3.4829618593157803, 3.482946100536598, 3.4830021317514666, 3.482986372972285, 3.4829776180949623, 3.4829583573648493, 3.4829741161440326, 3.482965361266708, 3.4829916258986793, 3.4829583573648493, 3.4829758671194972, 3.4829636102912445, 3.482967112242174, 3.482946100536597, 3.4829548554139205, 3.482982871021356, 3.482986372972286, 3.482968863217637], "Elapsed Time (ms)"=1322, "DMM Fault Array"=[FALSE, FALSE, FALSE, FALSE, FALSE, FALSE, FALSE, FALSE, FALSE, FALSE, FALSE, FALSE, FALSE, FALSE, FALSE, FALSE, FALSE, FALSE, FALSE, FALSE, FALSE, FALSE, FALSE, FALSE, FALSE, FALSE, FALSE, FALSE, FALSE, FALSE, FALSE, FALSE, FALSE, FALSE, FALSE, FALSE, FALSE, FALSE, FALSE, FALSE, FALSE, FALSE, FALSE, FALSE, FALSE, FALSE, FALSE, FALSE, FALSE, FALSE, FALSE, FALSE, FALSE, FALSE, FALSE, FALSE, FALSE, FALSE, FALSE, FALSE, FALSE, FALSE, FALSE, FALSE, FALSE, FALSE, FALSE, FALSE, FALSE, FALSE, FALSE, FALSE, FALSE, FALSE, FALSE, FALSE, FALSE, FALSE, FALSE, FALSE, FALSE, FALSE, FALSE, FALSE, FALSE, FALSE, FALSE, FALSE, FALSE, FALSE, FALSE, FALSE, FALSE, FALSE, FALSE, FALSE, FALSE, FALSE, FALSE, FALSE, FALSE, FALSE, FALSE, FALSE, FALSE, FALSE, FALSE, FALSE, FALSE, FALSE, FALSE, FALSE, FALSE, FALSE, FALSE, FALSE, FALSE, FALSE, FALSE, FALSE, FALSE, FALSE, FALSE, FALSE, FALSE, FALSE, FALSE, FALSE, FALSE, FALSE, FALSE, FALSE, FALSE, FALSE, FALSE, FALSE, FALSE, FALSE, FALSE, FALSE, FALSE, FALSE, FALSE, FALSE, FALSE, FALSE, FALSE, FALSE, FALSE, FALSE, FALSE, FALSE, FALSE, FALSE, FALSE, FALSE, FALSE, FALSE, FALSE, FALSE, FALSE, FALSE, FALSE, FALSE, FALSE, FALSE, FALSE, FALSE, FALSE, FALSE, FALSE, FALSE, FALSE, FALSE, FALSE, FALSE, FALSE, FALSE, FALSE, FALSE, FALSE, FALSE, FALSE, FALSE, FALSE, FALSE, FALSE, FALSE, FALSE, FALSE, FALSE, FALSE, FALSE, FALSE, FALSE, FALSE, FALSE, FALSE, FALSE, FALSE]}
  in  "5.5 Digit - 200 Measurements":T1={"V ch0 Array"=[3.4860206509621303, 3.486021645516196, 3.4860311540133595, 3.4860310587603, 3.486023466530679, 3.4860178550045133, 3.4860219732988074, 3.4860290724537326, 3.4860283412463815, 3.4860193650457525, 3.4860157874526876, 3.486021679134928, 3.486023850344497, 3.4860343085707566, 3.486020718199594, 3.4860140140647364, 3.4860208666823125, 3.486027884591974, 3.4860334989197033, 3.4860222786689277, 3.4860149946109953, 3.4860180539153256, 3.486027573618736, 3.486030302338898, 3.4860255620981158, 3.4860273410891875, 3.4860176925139914, 3.4860233796822993, 3.486030207085823, 3.486031714325511, 3.486023671044611, 3.4860149441828976, 3.486024186531795, 3.4860321121471407, 3.4860306581371083, 3.486018544188454, 3.4860139972553674, 3.48602242154853, 3.4860257666120544, 3.486034190905212], "V ch1 Array"=[3.4837797777764274, 3.4837820190250137, 3.4837711909927442, 3.483769689356184, 3.483768725619293, 3.483775807964846, 3.4837836299224443, 3.4837767380830167, 3.4837721351187145, 3.4837673556560866, 3.4837720398656487, 3.483781170152116, 3.483778278941426, 3.483768546319401, 3.4837630300463043, 3.4837706558946375, 3.483771406712918, 3.4837799346638194, 3.483773807650478, 3.483764968726334, 3.483767448107591, 3.483774409986043, 3.4837810216693965, 3.4837729895947427, 3.4837661397787243, 3.483767436901349, 3.4837759900663006, 3.4837824084419617, 3.483775261660506, 3.483768061649396, 3.4837662126193045, 3.483775082360619, 3.4837807191008348, 3.4837780296025196, 3.4837685155022315, 3.483768941339466, 3.4837718493595173, 3.483780161590247, 3.4837808535757526, 3.4837700143372263], "V ch2 Array"=[3.4809020201837573, 3.480894374724487, 3.4808826585974546, 3.4808894803978703, 3.480899467961918, 3.480901246952983, 3.4808979635237987, 3.4808945120009582, 3.4808907719173665, 3.4808957586954947, 3.4808997789351586, 3.4808924304413336, 3.480895257216119, 3.4808861997702394, 3.480897971928476, 3.480903689913961, 3.4808986190890145, 3.4808943971369697, 3.480883669960885, 3.4808941982261605, 3.480894545619691, 3.480896408657586, 3.4808919905962927, 3.4808856786799396, 3.480890399309793, 3.480896531926257, 3.480904000887204, 3.480893688342112, 3.4808883093454734, 3.4808868749463766, 3.4808981848471032, 3.4809015691324783, 3.480895593403411, 3.480892203514908, 3.480889491604113, 3.4808956438315057, 3.480908351711036, 3.4809015607277924, 3.480892901103528, 3.4808868553354517], "V ch3 Array"=[3.4846670516748333, 3.4846598432590365, 3.484666583814187, 3.4846684580583327, 3.484677109277905, 3.4846680714429494, 3.4846629613961473, 3.484665241866598, 3.4846723578308794, 3.48467922445627, 3.4846741116079065, 3.484665272683757, 3.4846627792947027, 3.484671472537691, 3.4846790227438897, 3.48467314226789, 3.4846727752634337, 3.4846644182077333, 3.4846717835109295, 3.484679585857604, 3.48467574211626, 3.484668007007045, 3.484657316251249, 3.4846709458442686, 3.484672831294646, 3.4846778488899415, 3.484668690587874, 3.4846608406146675, 3.4846649084808647, 3.4846697719903186, 3.4846774034417853, 3.4846725035120416, 3.4846617259078587, 3.48466402318767, 3.48467293495239, 3.484678524066083, 3.484672736041578, 3.4846637682456385, 3.484662625208856, 3.484673321567784], "V ch4 Array"=[3.482935712349363, 3.4829492550939922, 3.482951084513158, 3.482953331364872, 3.4829462518208767, 3.482937998422927, 3.4829462434161917, 3.4829482129133975, 3.482951384280159, 3.4829422371843344, 3.482936544412897, 3.4829448146202115, 3.482947823496449, 3.482957542110672, 3.482945643882191, 3.482937835932402, 3.4829397998264824, 3.4829489357160694, 3.4829584218007454, 3.4829471679312345, 3.48294719594685, 3.4829401780371874, 3.4829472827952306, 3.482959410751685, 3.4829556370493653, 3.4829448566436234, 3.4829407215399706, 3.4829451480059497, 3.482950081554416, 3.482957354406102, 3.4829469185923334, 3.482936479977, 3.4829420102579074, 3.4829464031051587, 3.482951860545487, 3.4829479663760554, 3.4829388052724206, 3.4829418505689493, 3.482950742722746, 3.4829575589200394], "Elapsed Time (ms)"=1418, "DMM Fault Array"=[FALSE, FALSE, FALSE, FALSE, FALSE, FALSE, FALSE, FALSE, FALSE, FALSE, FALSE, FALSE, FALSE, FALSE, FALSE, FALSE, FALSE, FALSE, FALSE, FALSE, FALSE, FALSE, FALSE, FALSE, FALSE, FALSE, FALSE, FALSE, FALSE, FALSE, FALSE, FALSE, FALSE, FALSE, FALSE, FALSE, FALSE, FALSE, FALSE, FALSE, FALSE, FALSE, FALSE, FALSE, FALSE, FALSE, FALSE, FALSE, FALSE, FALSE, FALSE, FALSE, FALSE, FALSE, FALSE, FALSE, FALSE, FALSE, FALSE, FALSE, FALSE, FALSE, FALSE, FALSE, FALSE, FALSE, FALSE, FALSE, FALSE, FALSE, FALSE, FALSE, FALSE, FALSE, FALSE, FALSE, FALSE, FALSE, FALSE, FALSE, FALSE, FALSE, FALSE, FALSE, FALSE, FALSE, FALSE, FALSE, FALSE, FALSE, FALSE, FALSE, FALSE, FALSE, FALSE, FALSE, FALSE, FALSE, FALSE, FALSE, FALSE, FALSE, FALSE, FALSE, FALSE, FALSE, FALSE, FALSE, FALSE, FALSE, FALSE, FALSE, FALSE, FALSE, FALSE, FALSE, FALSE, FALSE, FALSE, FALSE, FALSE, FALSE, FALSE, FALSE, FALSE, FALSE, FALSE, FALSE, FALSE, FALSE, FALSE, FALSE, FALSE, FALSE, FALSE, FALSE, FALSE, FALSE, FALSE, FALSE, FALSE, FALSE, FALSE, FALSE, FALSE, FALSE, FALSE, FALSE, FALSE, FALSE, FALSE, FALSE, FALSE, FALSE, FALSE, FALSE, FALSE, FALSE, FALSE, FALSE, FALSE, FALSE, FALSE, FALSE, FALSE, FALSE, FALSE, FALSE, FALSE, FALSE, FALSE, FALSE, FALSE, FALSE, FALSE, FALSE, FALSE, FALSE, FALSE, FALSE, FALSE, FALSE, FALSE, FALSE, FALSE, FALSE, FALSE, FALSE, FALSE, FALSE, FALSE, FALSE, FALSE, FALSE, FALSE, FALSE, FALSE, FALSE, FALSE, FALSE]}
  in  "6.5 Digit - 200 Measurements":T1={"V ch0 Array"=[3.486007276323045, 3.486007488486389, 3.4860073172085833, 3.48600778289756, 3.486007277066716, 3.48600704269229, 3.4860079889516267, 3.4860078053536183, 3.4860074724618775, 3.486007138864972, 3.4860066939855705, 3.4860067073494285, 3.4860081026328706, 3.4860067644334, 3.4860073555280358, 3.486006746645297, 3.4860071738385447, 3.486007186310952, 3.48600725370475, 3.4860066052991687, 3.486006257190876, 3.486006316381739, 3.4860069859057754, 3.486006134020886, 3.486005732796398, 3.486006033273634, 3.486005896848253, 3.4860058348558574, 3.486005886079627, 3.4860058053715766, 3.4860058155929083, 3.486006035777022, 3.4860064007526304, 3.4860053918354876, 3.486004794222689, 3.4860050773537794, 3.4860050350562255, 3.4860057407186464, 3.486005720021455, 3.486005038268717], "V ch1 Array"=[3.483756199353635, 3.483756553142396, 3.483756711647847, 3.4837572088816597, 3.48375692779987, 3.4837569971666453, 3.483756642511936, 3.4837561034881754, 3.483756037426233, 3.48375671197069, 3.4837559272523877, 3.4837565979711407, 3.4837555805775047, 3.483755433113611, 3.4837561159230783, 3.4837555015951227, 3.483755158280515, 3.483756825695055, 3.483755601088368, 3.483755115106389, 3.4837555849625086, 3.483754975382758, 3.483755448118047, 3.4837546227885174, 3.483754912467896, 3.4837552220678574, 3.483755666743301, 3.4837553824311556, 3.483754706126229, 3.483754927291571, 3.483754753491377, 3.483754398895731, 3.48375474272133, 3.483754969845828, 3.48375408399525, 3.48375462482431, 3.4837542959016226, 3.4837553363146583, 3.4837542012388902, 3.4837546597684823], "V ch2 Array"=[3.4808810457410573, 3.4808812929163633, 3.4808808002413936, 3.4808806745512713, 3.4808812103208298, 3.4808812143297807, 3.4808806620375643, 3.4808802056238903, 3.4808797728494074, 3.4808811012331367, 3.480879433958281, 3.4808793142371366, 3.480878669930749, 3.4808793789167716, 3.4808785832577627, 3.4808783140012585, 3.480877944514941, 3.4808782565470624, 3.4808779185845915, 3.4808775062178894, 3.4808768336750346, 3.480877377840251, 3.4808764388454327, 3.4808777526806165, 3.4808765504816748, 3.480877766532824, 3.4808764236460346, 3.4808764661468627, 3.480876139975534, 3.4808756196171355, 3.4808755983940993, 3.480875242392487, 3.480876068778303, 3.480875408450911, 3.4808748825400992, 3.4808748097219686, 3.48087500297719, 3.4808752841218125, 3.480874985372623, 3.4808741408140937], "V ch3 Array"=[3.484656289005541, 3.4846560008441743, 3.484656615282902, 3.484655957764772, 3.4846558086282267, 3.4846558734638053, 3.4846557080367826, 3.484655303529688, 3.484655499138367, 3.484655411504402, 3.4846550658444753, 3.4846550013963715, 3.48465451472455, 3.4846543043778806, 3.48465339269957, 3.4846541844814176, 3.4846533321251676, 3.4846540710961444, 3.4846535638228944, 3.4846522395828106, 3.4846527451616027, 3.484652446319622, 3.4846527202903763, 3.4846518185455593, 3.484652001298707, 3.484652321137677, 3.484651480337147, 3.4846511320023175, 3.4846509773745447, 3.4846505387415254, 3.4846506392876098, 3.4846509382168462, 3.484650517640251, 3.484649642191482, 3.4846509479500116, 3.484650195167144, 3.484650477362746, 3.4846491268155217, 3.48464861471377, 3.4846497184895195], "V ch4 Array"=[3.482933771868285, 3.482933246370093, 3.482934112822907, 3.4829333948874215, 3.4829332440536778, 3.4829330074621287, 3.482932860767126, 3.4829325322114975, 3.4829319317332255, 3.4829324168896654, 3.4829317859084163, 3.482930969217602, 3.4829313529196697, 3.4829312433362456, 3.482931480065567, 3.4829307742951103, 3.4829315988613185, 3.482930911301376, 3.482931839131908, 3.4829309098851513, 3.4829308118494944, 3.4829296611124922, 3.4829299159103413, 3.482930796524262, 3.482930218468753, 3.482931454621633, 3.4829311379286483, 3.48293005365676, 3.4829305062832887, 3.482929861623295, 3.4829289899842655, 3.4829312017095186, 3.48292957741501, 3.482930186248675, 3.4829281737352176, 3.482929605619413, 3.4829290532156088, 3.4829289676487702, 3.482929246736649, 3.482928618591218], "Elapsed Time (ms)"=57590, "DMM Fault Array"=[FALSE, FALSE, FALSE, FALSE, FALSE, FALSE, FALSE, FALSE, FALSE, FALSE, FALSE, FALSE, FALSE, FALSE, FALSE, FALSE, FALSE, FALSE, FALSE, FALSE, FALSE, FALSE, FALSE, FALSE, FALSE, FALSE, FALSE, FALSE, FALSE, FALSE, FALSE, FALSE, FALSE, FALSE, FALSE, FALSE, FALSE, FALSE, FALSE, FALSE, FALSE, FALSE, FALSE, FALSE, FALSE, FALSE, FALSE, FALSE, FALSE, FALSE, FALSE, FALSE, FALSE, FALSE, FALSE, FALSE, FALSE, FALSE, FALSE, FALSE, FALSE, FALSE, FALSE, FALSE, FALSE, FALSE, FALSE, FALSE, FALSE, FALSE, FALSE, FALSE, FALSE, FALSE, FALSE, FALSE, FALSE, FALSE, FALSE, FALSE, FALSE, FALSE, FALSE, FALSE, FALSE, FALSE, FALSE, FALSE, FALSE, FALSE, FALSE, FALSE, FALSE, FALSE, FALSE, FALSE, FALSE, FALSE, FALSE, FALSE, FALSE, FALSE, FALSE, FALSE, FALSE, FALSE, FALSE, FALSE, FALSE, FALSE, FALSE, FALSE, FALSE, FALSE, FALSE, FALSE, FALSE, FALSE, FALSE, FALSE, FALSE, FALSE, FALSE, FALSE, FALSE, FALSE, FALSE, FALSE, FALSE, FALSE, FALSE, FALSE, FALSE, FALSE, FALSE, FALSE, FALSE, FALSE, FALSE, FALSE, FALSE, FALSE, FALSE, FALSE, FALSE, FALSE, FALSE, FALSE, FALSE, FALSE, FALSE, FALSE, FALSE, FALSE, FALSE, FALSE, FALSE, FALSE, FALSE, FALSE, FALSE, FALSE, FALSE, FALSE, FALSE, FALSE, FALSE, FALSE, FALSE, FALSE, FALSE, FALSE, FALSE, FALSE, FALSE, FALSE, FALSE, FALSE, FALSE, FALSE, FALSE, FALSE, FALSE, FALSE, FALSE, FALSE, FALSE, FALSE, FALSE, FALSE, FALSE, FALSE, FALSE, FALSE, FALSE, FALSE, FALSE, FALSE, FALSE, FALSE]}
  in  "7.5 Digit - 200 Measurements":T1={"V ch0 Array"=[3.4860085618860106, 3.486008590626267, 3.486008340598651, 3.4860079967103563, 3.4860067307869147, 3.4860065165631084, 3.486005774745495, 3.4860055816695668, 3.486006006962822, 3.4860053059676575, 3.486005567774427, 3.4860057089775314, 3.486005925467364, 3.486005280650062, 3.4860053026162987, 3.486004543856078, 3.486005005123501, 3.486005354248964, 3.486004989400345, 3.48600468532152, 3.486005155323255, 3.486005173573889, 3.486004948458652, 3.4860046275785495, 3.4860048944598896, 3.486004850458057, 3.486004498378284, 3.4860048195735653, 3.486004127492709, 3.486004531561373, 3.486004835753217, 3.486004431737616, 3.4860040810025654, 3.4860040316168046, 3.486003572804981, 3.4860038517480487, 3.486003067966893, 3.4860042541364527, 3.4860043300701133, 3.48600418843923], "V ch1 Array"=[3.483759152743593, 3.4837585250939904, 3.4837579648896306, 3.4837574507074054, 3.4837568509614094, 3.4837562791303744, 3.4837551011489345, 3.483755039614413, 3.4837553943356454, 3.483755398297787, 3.4837545863610657, 3.483754443468955, 3.48375458488637, 3.4837541520402766, 3.483754367679233, 3.4837538615354724, 3.4837536942543985, 3.4837530549864657, 3.483753359898949, 3.483753094214852, 3.4837530565103796, 3.48375287360835, 3.4837531561746555, 3.4837528453062565, 3.4837525836136485, 3.4837528332992527, 3.4837519932826155, 3.4837525631090918, 3.483752484263212, 3.483752366886127, 3.4837530533532335, 3.4837527163243034, 3.483752186044433, 3.4837514040762323, 3.483751820823942, 3.4837515280604276, 3.483751516722055, 3.4837516592551543, 3.483752326088813, 3.4837514933716536], "V ch2 Array"=[3.4808830130096347, 3.4808821849398854, 3.4808813111553474, 3.4808808220531846, 3.480879615833457, 3.4808782076132854, 3.480877466636017, 3.480877341223312, 3.480877568610515, 3.480876860943647, 3.480876205861217, 3.480875821494147, 3.480875838670589, 3.480876065846462, 3.4808752556519855, 3.4808748402944825, 3.480874108259076, 3.48087394988443, 3.4808737868551427, 3.480873705791051, 3.480874113709122, 3.4808737910127006, 3.4808734844161995, 3.4808734869166624, 3.4808732409302117, 3.4808729972612626, 3.4808728933554556, 3.4808725294173004, 3.480872330092393, 3.4808726651389494, 3.480872942484635, 3.4808721640402114, 3.4808725036408514, 3.480871670101209, 3.480872029968027, 3.480871640465131, 3.4808721312208615, 3.480872372941337, 3.480872208217519, 3.4808724147703365], "V ch3 Array"=[3.484659439519947, 3.484658551926035, 3.484657898303126, 3.484656957864823, 3.4846555951370295, 3.4846542820101627, 3.4846540742799044, 3.48465414098835, 3.484653365586936, 3.4846529391945245, 3.4846517267123263, 3.4846521530638506, 3.4846518198364977, 3.484652141590008, 3.4846522374828304, 3.484651215929581, 3.4846509640349987, 3.4846504822125626, 3.48465057293914, 3.4846509551405305, 3.4846505907500935, 3.484650871427114, 3.484650211223542, 3.484650587144478, 3.484650469373251, 3.4846502923058793, 3.4846505192593744, 3.484650108268589, 3.484650018976092, 3.484650329977102, 3.484650228735876, 3.4846492337208095, 3.4846485782113823, 3.4846482941660795, 3.4846485116793238, 3.4846483071760415, 3.4846482507618237, 3.4846490501378646, 3.4846490374578316, 3.4846489124479634], "V ch4 Array"=[3.482935584623865, 3.4829353704429806, 3.482935185556424, 3.4829344648974025, 3.482933544177533, 3.4829325906882964, 3.482932315633546, 3.4829323020174896, 3.482932296204778, 3.48293171954385, 3.482931254865685, 3.482931069760455, 3.4829312406514426, 3.4829312719445102, 3.4829315160538643, 3.4829307368694598, 3.4829304247233477, 3.4829304967775663, 3.482929817249088, 3.482930315710686, 3.4829297317702346, 3.4829297627120255, 3.482929997313331, 3.48293028781108, 3.4829299552764734, 3.4829299974655816, 3.482930364285701, 3.4829305519833875, 3.482930250818271, 3.482930206232788, 3.4829296020363225, 3.482929382751545, 3.482929504612687, 3.4829292237285507, 3.482928922246743, 3.4829283194885328, 3.4829285266292036, 3.4829283393581707, 3.4829286277392755, 3.4829283621794787], "Elapsed Time (ms)"=227179, "DMM Fault Array"=[FALSE, FALSE, FALSE, FALSE, FALSE, FALSE, FALSE, FALSE, FALSE, FALSE, FALSE, FALSE, FALSE, FALSE, FALSE, FALSE, FALSE, FALSE, FALSE, FALSE, FALSE, FALSE, FALSE, FALSE, FALSE, FALSE, FALSE, FALSE, FALSE, FALSE, FALSE, FALSE, FALSE, FALSE, FALSE, FALSE, FALSE, FALSE, FALSE, FALSE, FALSE, FALSE, FALSE, FALSE, FALSE, FALSE, FALSE, FALSE, FALSE, FALSE, FALSE, FALSE, FALSE, FALSE, FALSE, FALSE, FALSE, FALSE, FALSE, FALSE, FALSE, FALSE, FALSE, FALSE, FALSE, FALSE, FALSE, FALSE, FALSE, FALSE, FALSE, FALSE, FALSE, FALSE, FALSE, FALSE, FALSE, FALSE, FALSE, FALSE, FALSE, FALSE, FALSE, FALSE, FALSE, FALSE, FALSE, FALSE, FALSE, FALSE, FALSE, FALSE, FALSE, FALSE, FALSE, FALSE, FALSE, FALSE, FALSE, FALSE, FALSE, FALSE, FALSE, FALSE, FALSE, FALSE, FALSE, FALSE, FALSE, FALSE, FALSE, FALSE, FALSE, FALSE, FALSE, FALSE, FALSE, FALSE, FALSE, FALSE, FALSE, FALSE, FALSE, FALSE, FALSE, FALSE, FALSE, FALSE, FALSE, FALSE, FALSE, FALSE, FALSE, FALSE, FALSE, FALSE, FALSE, FALSE, FALSE, FALSE, FALSE, FALSE, FALSE, FALSE, FALSE, FALSE, FALSE, FALSE, FALSE, FALSE, FALSE, FALSE, FALSE, FALSE, FALSE, FALSE, FALSE, FALSE, FALSE, FALSE, FALSE, FALSE, FALSE, FALSE, FALSE, FALSE, FALSE, FALSE, FALSE, FALSE, FALSE, FALSE, FALSE, FALSE, FALSE, FALSE, FALSE, FALSE, FALSE, FALSE, FALSE, FALSE, FALSE, FALSE, FALSE, FALSE, FALSE, FALSE, FALSE, FALSE, FALSE, FALSE, FALSE, FALSE, FALSE, FALSE, FALSE, FALSE, FALSE, FALSE]}
  in  "7.5 Digit - All Channels 2":T1={"V ch0 Array"=[3.4860091405631297, 3.486009109359947, 3.48600818671822, 3.4860076325339744, 3.486006849105656, 3.4860066251627297, 3.4860061215719806, 3.486005989728432], "V ch1 Array"=[3.4837607383453433, 3.4837601411863166, 3.4837597083911276, 3.4837591982574185, 3.483758164664129, 3.48375688618012, 3.4837562560353597, 3.483756287818867], "V ch2 Array"=[3.4808838859960334, 3.4808831039389716, 3.480882191398215, 3.480880686409241, 3.480879941214358, 3.4808791419777383, 3.4808785918129796, 3.480878498788436], "V ch3 Array"=[3.484661264804309, 3.4846607916763306, 3.48466055498231, 3.4846598870164707, 3.484658337082086, 3.4846577504168854, 3.4846567698725113, 3.484655717462156], "V ch4 Array"=[3.482935896793945, 3.482935692335635, 3.482934549804364, 3.4829339013538423, 3.4829332799487647, 3.482932613692898, 3.482932424648914, 3.482932125266278], "Elapsed Time (ms)"=46115, "DMM Fault Array"=[FALSE, FALSE, FALSE, FALSE, FALSE, FALSE, FALSE, FALSE, FALSE, FALSE, FALSE, FALSE, FALSE, FALSE, FALSE, FALSE, FALSE, FALSE, FALSE, FALSE, FALSE, FALSE, FALSE, FALSE, FALSE, FALSE, FALSE, FALSE, FALSE, FALSE, FALSE, FALSE, FALSE, FALSE, FALSE, FALSE, FALSE, FALSE, FALSE, FALSE]}
  in  "7.5 Digit - All Channels":T1={"V ch0 Array"=[3.4860112019011575, 3.4860106719629336, 3.4860096022940508, 3.4860091404359883, 3.4860088355110253, 3.486007924623058, 3.4860078606179856, 3.4860071112809696], "V ch1 Array"=[3.483765397997347, 3.483765011849362, 3.483763829347856, 3.4837629547082987, 3.483762942133045, 3.483762664227104, 3.483762271114208, 3.483761709190893], "V ch2 Array"=[3.4808884619064338, 3.4808873278157675, 3.48088643364081, 3.4808849391728103, 3.480884344991334, 3.4808836336156683, 3.480882943307825, 3.4808831990607096], "V ch3 Array"=[3.4846662264354107, 3.4846664120627953, 3.4846654613390764, 3.484664750779259, 3.4846636539869054, 3.484662171539861, 3.4846616457943353, 3.484661150300191], "V ch4 Array"=[3.4829357656945183, 3.4829355599883214, 3.4829351239537516, 3.4829345126487596, 3.4829349784257846, 3.4829343331131577, 3.4829344429417315, 3.4829344448605513], "Elapsed Time (ms)"=46121, "DMM Fault Array"=[FALSE, FALSE, FALSE, FALSE, FALSE, FALSE, FALSE, FALSE, FALSE, FALSE, FALSE, FALSE, FALSE, FALSE, FALSE, FALSE, FALSE, FALSE, FALSE, FALSE, FALSE, FALSE, FALSE, FALSE, FALSE, FALSE, FALSE, FALSE, FALSE, FALSE, FALSE, FALSE, FALSE, FALSE, FALSE, FALSE, FALSE, FALSE, FALSE, FALSE]}
  in  "7.5 Digit Automated ch0 only":T1={"V ch0 Array"=[3.48601076737072, 3.4860101864392146, 3.4860102136104922, 3.48601071941728, 3.4860113841698475, 3.486012105978004, 3.486012884805511, 3.4860131080501287], "V ch1 Array"=[3.486009902856364, 3.486009642081732, 3.4860104195933355, 3.486010500318132, 3.486011261927736, 3.4860117860949282, 3.4860126402823632, 3.4860134532317852], "V ch2 Array"=[3.4860096571438257, 3.4860099899410724, 3.486010901405744, 3.486011066051613, 3.486011384907023, 3.486012303315762, 3.4860130197253634, 3.486013628422841], "V ch3 Array"=[3.4860096356996637, 3.486010161566699, 3.4860107596410854, 3.4860110405776688, 3.486011557288925, 3.4860128857632713, 3.4860133153836173, 3.4860134628956634], "V ch4 Array"=[3.4860098669347566, 3.486010509789506, 3.4860108140085275, 3.4860111601743675, 3.4860118454750415, 3.4860124865680344, 3.486013135089857, 3.4860134413362323], "Elapsed Time (ms)"=46326, "DMM Fault Array"=[FALSE, FALSE, FALSE, FALSE, FALSE, FALSE, FALSE, FALSE, FALSE, FALSE, FALSE, FALSE, FALSE, FALSE, FALSE, FALSE, FALSE, FALSE, FALSE, FALSE, FALSE, FALSE, FALSE, FALSE, FALSE, FALSE, FALSE, FALSE, FALSE, FALSE, FALSE, FALSE, FALSE, FALSE, FALSE, FALSE, FALSE, FALSE, FALSE, FALSE]}
  in  "7.5 Digit Manual Results":T1={"V ch0 Array"=[3.4860192438984856, 3.4860191297168432, 3.4860192480889696, 3.486019388780445, 3.4860200552848166, 3.4860195698501135, 3.4860194367740833, 3.48601943363801, 3.4860193560307953, 3.4860188399429166, 3.486019346172368, 3.4860197228808754, 3.4860192492604813, 3.4860198681823347, 3.486019386629169, 3.486019609000733, 3.4860194222252203, 3.486019475094303, 3.4860195777883813, 3.4860198327972123, 3.4860194844791064, 3.4860192846597724, 3.486019604192855, 3.4860193890850635, 3.486019882549224, 3.4860193407836872, 3.486019819402258, 3.4860195718672933, 3.486019850290971, 3.486020065378193, 3.4860200812401376, 3.486019332827698, 3.486019539704669, 3.4860191856958327, 3.486019603338049, 3.4860197214840167, 3.4860195162856176, 3.486019661979488, 3.4860196152518625, 3.48601960972234, 3.486019510427399, 3.4860193955138996, 3.486019403923719, 3.4860191116981416, 3.486019283259686, 3.48601881184557, 3.4860196673230894, 3.486018902499217, 3.486019173963923, 3.486019332419299, 3.486019671202645, 3.486019499160391, 3.4860193137480726, 3.4860193110217956, 3.4860195130088014, 3.486019457464569, 3.486018832088054, 3.4860192806634824, 3.486019456596911, 3.4860193546431457, 3.486019205666364, 3.4860194794988364, 3.486019332920187, 3.4860189764454312, 3.4860194155707083, 3.486019464342129, 3.486019459378369, 3.4860192395365615, 3.486019018887167, 3.4860187312440396, 3.4860194234856827, 3.486019167144491, 3.486019322954545, 3.48601941556311, 3.486019112865338, 3.4860191373093796, 3.4860190631335772, 3.4860189837060633, 3.486019421078644, 3.4860195807691094, 3.486018781084102, 3.4860192815150843, 3.4860191116507178, 3.4860196897391127, 3.486019054482244, 3.4860193237434984, 3.4860194341181536, 3.486019107534501, 3.486019323345851, 3.486019194973677, 3.486019161730881, 3.486019175960558, 3.4860194881647844, 3.486019137883692, 3.4860194237810673, 3.486019240702601, 3.4860195063002863, 3.4860195279338497, 3.48601941521367, 3.4860192998594033], "V ch1 Array"=[3.4837635496144497, 3.4837633047078356, 3.483763519496143, 3.4837638386501917, 3.4837636749838783, 3.4837637622882767, 3.4837639960874567, 3.4837640653526893, 3.4837639002914216, 3.4837639948081716, 3.483764380840748, 3.4837637486370903, 3.4837636058739494, 3.4837640082997314, 3.4837639377349143, 3.483764152676197, 3.483764186328907, 3.483763658922308, 3.483763950595508, 3.483764349614305, 3.4837638707197667, 3.4837639694240075, 3.483763685524895, 3.4837640426104857, 3.483763773323028, 3.483763498861096, 3.48376386163464, 3.483763856182671, 3.4837637805094976, 3.483763376025008, 3.483763485394124, 3.483763737216476, 3.4837637488823647, 3.4837636870799384, 3.48376348307593, 3.4837637531514787, 3.4837640725319123, 3.4837636718839913, 3.4837640882494845, 3.483763595720128, 3.4837638710640184, 3.4837634353037403, 3.4837640127310228, 3.483763765786545, 3.483763965435208, 3.4837639356094123, 3.483763874493519, 3.4837639386973054, 3.483763836392622, 3.4837635278265235, 3.4837637173072933, 3.4837639264438756, 3.483763640566874, 3.483763106913948, 3.4837632637092986, 3.4837636505867873, 3.483763618410148, 3.483763671849778, 3.4837632178283666, 3.483763387233682, 3.483763281131254, 3.4837636013322024, 3.4837633057079733, 3.483763227327618, 3.4837634820027947, 3.4837631861156715, 3.483762983477066, 3.4837630334263046, 3.48376290875784, 3.483763232599418, 3.483762992554408, 3.4837626856166883, 3.4837631059287872, 3.483762813425183, 3.4837629087040725, 3.4837626099036934, 3.4837629622175927, 3.48376292288895, 3.4837632589985734, 3.483762886524989, 3.4837632610144427, 3.483762640667348, 3.4837627900286097, 3.4837628605073703, 3.4837625301098667, 3.483762589933555, 3.483762644047744, 3.4837630383446054, 3.4837628475429008, 3.4837633574684297, 3.4837628873032394, 3.4837626059584355, 3.483762748980832, 3.4837627125543214, 3.4837627065039456, 3.4837625152019323, 3.483762655577027, 3.4837625644890657, 3.483762586641063, 3.4837624149674027], "V ch2 Array"=[3.480869179811629, 3.4808692218497557, 3.480869138671519, 3.480869054699297, 3.480869011510365, 3.480869157197732, 3.4808692155328744, 3.480869471635288, 3.4808689594292206, 3.48086945076089, 3.480869460297174, 3.480869073256913, 3.4808692935975163, 3.4808692152632608, 3.4808692867089013, 3.4808692057176573, 3.4808687717598494, 3.4808694889465652, 3.4808697225710654, 3.4808695479967744, 3.4808689900519267, 3.4808689501574617, 3.4808694493861148, 3.480869392710721, 3.4808696704117006, 3.480869061775111, 3.480869230832857, 3.4808690498110715, 3.480869272251721, 3.480869182984733, 3.480868986153201, 3.4808695148516193, 3.480869285336756, 3.480869113289467, 3.480869321219842, 3.4808696853476415, 3.4808695734255553, 3.480869235137222, 3.480869247933297, 3.4808693725489355, 3.4808693970987883, 3.480869510249631, 3.480869077447023, 3.480869142955564, 3.480869810198066, 3.4808695210330862, 3.4808690281746526, 3.4808697940447284, 3.4808695256214586, 3.480869543704313, 3.4808695752111873, 3.4808694743349164, 3.480869402997512, 3.4808696440759235, 3.480869426102383, 3.480869437921433, 3.480869608329062, 3.4808695813646384, 3.480869231247081, 3.480869681482936, 3.4808696850419185, 3.480869147852085, 3.480869498009006, 3.480869210180875, 3.4808695475881706, 3.4808691625176307, 3.480869831997257, 3.4808697720708257, 3.4808697676147338, 3.4808693613028483, 3.480869321113382, 3.4808695723953145, 3.4808696503256313, 3.480869784646468, 3.4808693231656824, 3.480869815348858, 3.4808695842415895, 3.480870030556013, 3.4808698084316507, 3.480869756575092, 3.4808700398397106, 3.480869601892204, 3.4808695224207016, 3.480870206481561, 3.4808697521028567, 3.4808696686542224, 3.4808694863409126, 3.4808695575238113, 3.4808699065023303, 3.4808699638400196, 3.4808698631823836, 3.4808701101021295, 3.480869576271954, 3.4808697499119545, 3.480870271581758, 3.480869580700272, 3.4808700517526905, 3.4808702583002464, 3.4808700507095285, 3.480869823475541], "V ch3 Array"=[3.4846462570940635, 3.484646344612051, 3.484645744648206, 3.484645912481853, 3.4846463765223765, 3.4846459790344033, 3.484645991388148, 3.4846459949495276, 3.4846461321623687, 3.4846459792980466, 3.4846459502897926, 3.484645900398946, 3.484646406044855, 3.484646675084715, 3.4846462272866976, 3.484646061071726, 3.4846463560563388, 3.4846458628621204, 3.484646481637977, 3.484646699310659, 3.4846463490174218, 3.4846461232936154, 3.4846460582414216, 3.4846463570899213, 3.4846459057947308, 3.4846460556842596, 3.484646296030384, 3.4846460469738423, 3.48464658781997, 3.4846460245693365, 3.4846462795314737, 3.484646537085635, 3.4846463696141208, 3.4846462323319045, 3.4846461621354017, 3.484646601971744, 3.484646588329547, 3.484646695791384, 3.4846460264137344, 3.4846461593422626, 3.4846466656982935, 3.484646823450527, 3.484647012524444, 3.4846463505570626, 3.4846467729305797, 3.484646413280307, 3.48464649989975, 3.48464616810511, 3.4846465502016866, 3.4846468176917242, 3.484646635790896, 3.4846464989218693, 3.4846463465061155, 3.4846469659954202, 3.484647055263412, 3.484646589351149, 3.4846465424842292, 3.4846469626004875, 3.4846465155978295, 3.484646895602941, 3.4846462809210985, 3.4846465125913824, 3.4846467493560573, 3.4846468222999647, 3.4846468884980775, 3.4846465504399218, 3.4846466232460154, 3.484646653097931, 3.4846467313351366, 3.484646901512995, 3.4846468026062616, 3.4846468641960726, 3.4846469829861624, 3.4846471909486487, 3.484646883370365, 3.4846465532654762, 3.484647151525274, 3.484647178327674, 3.484646970005987, 3.4846469124260966, 3.4846470266927594, 3.484646758486475, 3.484646811518315, 3.484646952996467, 3.4846469195374183, 3.484647335077417, 3.4846469162977516, 3.484646966685987, 3.484646746192782, 3.4846472376848387, 3.4846470826060396, 3.484646707902158, 3.4846471664925933, 3.4846471496125684, 3.484646829256042, 3.4846473259364736, 3.484647176634124, 3.4846472224270593, 3.4846474931875475, 3.4846470047324956], "V ch4 Array"=[3.482921883101798, 3.48292201038743, 3.482921963650252, 3.48292232595166, 3.4829219295743936, 3.4829222500251023, 3.4829218631289827, 3.482921530631896, 3.4829218244984688, 3.4829222060011986, 3.482921953922925, 3.482922434358391, 3.4829218861123223, 3.4829224024812797, 3.482922119408693, 3.482921891932435, 3.482922097428749, 3.4829221620547077, 3.4829221751564283, 3.482922233556675, 3.4829222935528996, 3.482922460577868, 3.482922010835762, 3.4829223716134146, 3.4829219243006335, 3.482921971962534, 3.48292214332319, 3.4829226800188824, 3.482922110730465, 3.482922308133039, 3.4829222890143448, 3.4829218963348003, 3.4829222321373243, 3.4829224166371646, 3.482922437339793, 3.4829227251192765, 3.4829224629498805, 3.4829224981761575, 3.482922744640211, 3.482922055871053, 3.482922617234262, 3.4829224386727837, 3.4829223546749937, 3.4829226079428963, 3.4829226019926987, 3.482922626244296, 3.482923102428407, 3.4829225941259927, 3.482922684262713, 3.482922875117361, 3.482922843526534, 3.4829228813035367, 3.482922798160215, 3.4829228033313098, 3.482922729208571, 3.4829230463638323, 3.482923001878261, 3.4829225660015597, 3.4829227170501635, 3.482922912556587, 3.482923170700634, 3.482922745453038, 3.4829229565113202, 3.482922859113936, 3.482922615231731, 3.482923042810891, 3.482922931359675, 3.4829233142114684, 3.482922846410176, 3.482923004292494, 3.48292354951055, 3.482923184798173, 3.4829227918015793, 3.482923015660196, 3.4829232528293685, 3.4829227291783544, 3.4829230564932825, 3.482922959508547, 3.4829228878182956, 3.4829230996323073, 3.4829230305207095, 3.482922900213177, 3.482923542767866, 3.482923191269675, 3.4829231627478645, 3.482923425303535, 3.482923253521273, 3.482923128067224, 3.482923205492421, 3.4829229699938544, 3.482923351524313, 3.4829234043244677, 3.4829230246211997, 3.482923045679957, 3.4829234300085905, 3.4829232984556935, 3.4829235896745185, 3.482923548361324, 3.48292348716183, 3.482923770747649], "Elapsed Time (ms)"=11164, "DMM Fault Array"=[]}
  in  "Results":T1={"V ch0 Array"=[2.6402355104591723e-06, 3.2050422226470716e-06, 3.2738385547093894e-06, 3.0004056082675545e-06, 3.190429018678622e-06, 3.265655292871135e-06, 3.4283206777974678e-06], "V ch1 Array"=[3.579181433209794e-06, 3.538102305000126e-06, 3.3674070559982216e-06, 3.2951997357567907e-06, 3.0614196043446336e-06, 3.247982674682344e-06, 3.4582756481500834e-06], "V ch2 Array"=[2.636942617106564e-06, 2.444215695573972e-06, 2.3600385872845126e-06, 2.3785120159418297e-06, 2.39158079459529e-06, 2.5415574149365358e-06, 2.629696833600491e-06], "V ch3 Array"=[4.29015971742814e-06, 4.582682915243894e-06, 4.199947801068903e-06, 4.210565880465411e-06, 4.1249236933492e-06, 4.3283146693326225e-06], "V ch4 Array"=[3.2068632920738282e-06, 3.2352868353418705e-06, 3.218523090660476e-06, 3.1985005992771743e-06, 3.2252632419667723e-06, 3.3472279144313767e-06], "Elapsed Time (ms)"=11164, "DMM Fault Array"=[]}
  out "ch4 range":dbl=5.939087689643685e-06 format="%#_6p"
  out "ch4 std dev":dbl=1.4806985631333817e-06 format="%#.3p"
  out "ch4 mean":dbl=3.4829310355717924 format="%#.6p"
  out "Histogram Graph ch4":T2(graph)={"X Values"=[3.482928470689602, 3.482929064598371, 3.48292965850714, 3.4829302524159087, 3.4829308463246775, 3.4829314402334464, 3.482932034142215, 3.482932628050984, 3.482933221959753, 3.4829338158685217], "Histogram: h(x)"=[2, 4, 5, 4, 7, 6, 3, 3, 4, 2]}
  out "ch3 range":dbl=8.000569132082802e-06 format="%#_6p"
  out "ch3 std dev":dbl=2.281539089930446e-06 format="%#.3p"
  out "ch3 mean":dbl=3.484652928409848 format="%#.6p"
  out "Histogram Graph ch3":T2(graph)={"X Values"=[3.4846490147422267, 3.48464981479914, 3.484650614856053, 3.484651414912966, 3.4846522149698793, 3.4846530150267925, 3.4846538150837056, 3.484654615140619, 3.484655415197532, 3.484656215254445], "Histogram: h(x)"=[2, 3, 7, 2, 5, 4, 3, 3, 6, 5]}
  out "ch2 range":dbl=7.152102269536442e-06 format="%#_6p"
  out "ch2 std dev":dbl=2.1806636220050264e-06 format="%#.3p"
  out "ch2 mean":dbl=3.4808778023254034 format="%#.6p"
  out "Histogram Graph ch2":T2(graph)={"X Values"=[3.4808744984192073, 3.4808752136294343, 3.4808759288396613, 3.4808766440498884, 3.4808773592601154, 3.4808780744703425, 3.4808787896805695, 3.4808795048907966, 3.4808802201010236, 3.4808809353112506], "Histogram: h(x)"=[2, 6, 4, 5, 2, 6, 2, 4, 1, 8]}
  out "ch1 range":dbl=3.124886409633376e-06 format="%#_6p"
  out "ch1 std dev":dbl=8.542956909478713e-07 format="%#.3p"
  out "ch1 mean":dbl=3.48375553663424 format="%#.6p"
  out "Histogram Graph ch1":T2(graph)={"X Values"=[3.4837542402395707, 3.483754552728212, 3.483754865216853, 3.4837551777054943, 3.4837554901941354, 3.4837558026827766, 3.483756115171418, 3.483756427660059, 3.4837567401487, 3.4837570526373414], "Histogram: h(x)"=[3, 5, 6, 3, 8, 2, 4, 1, 5, 3]}
  out "ch0 range":dbl=3.3084101818126044e-06 format="%#_6p"
  out "ch0 std dev":dbl=8.7047897478175e-07 format="%#.3p"
  out "ch0 mean":dbl=3.4860065278089722 format="%#.6p"
  out "Histogram Graph ch0":T2(graph)={"X Values"=[3.486004959643198, 3.4860052904842163, 3.4860056213252344, 3.4860059521662525, 3.4860062830072707, 3.486006613848289, 3.486006944689307, 3.486007275530325, 3.486007606371343, 3.4860079372123614], "Histogram: h(x)"=[4, 1, 3, 7, 4, 5, 2, 8, 2, 4]}
  out "Waveform Chart ch1":dbl[](graph)=[3.483756199353635, 3.483756553142396, 3.483756711647847, 3.4837572088816597, 3.48375692779987, 3.4837569971666453, 3.483756642511936, 3.4837561034881754, 3.483756037426233, 3.48375671197069, 3.4837559272523877, 3.4837565979711407, 3.4837555805775047, 3.483755433113611, 3.4837561159230783, 3.4837555015951227, 3.483755158280515, 3.483756825695055, 3.483755601088368, 3.483755115106389, 3.4837555849625086, 3.483754975382758, 3.483755448118047, 3.4837546227885174, 3.483754912467896, 3.4837552220678574, 3.483755666743301, 3.4837553824311556, 3.483754706126229, 3.483754927291571, 3.483754753491377, 3.483754398895731, 3.48375474272133, 3.483754969845828, 3.48375408399525, 3.48375462482431, 3.4837542959016226, 3.4837553363146583, 3.4837542012388902, 3.4837546597684823]
  out "Waveform Chart ch4":dbl[](graph)=[3.482933771868285, 3.482933246370093, 3.482934112822907, 3.4829333948874215, 3.4829332440536778, 3.4829330074621287, 3.482932860767126, 3.4829325322114975, 3.4829319317332255, 3.4829324168896654, 3.4829317859084163, 3.482930969217602, 3.4829313529196697, 3.4829312433362456, 3.482931480065567, 3.4829307742951103, 3.4829315988613185, 3.482930911301376, 3.482931839131908, 3.4829309098851513, 3.4829308118494944, 3.4829296611124922, 3.4829299159103413, 3.482930796524262, 3.482930218468753, 3.482931454621633, 3.4829311379286483, 3.48293005365676, 3.4829305062832887, 3.482929861623295, 3.4829289899842655, 3.4829312017095186, 3.48292957741501, 3.482930186248675, 3.4829281737352176, 3.482929605619413, 3.4829290532156088, 3.4829289676487702, 3.482929246736649, 3.482928618591218]
  out "Waveform Chart ch2":dbl[](graph)=[3.4808810457410573, 3.4808812929163633, 3.4808808002413936, 3.4808806745512713, 3.4808812103208298, 3.4808812143297807, 3.4808806620375643, 3.4808802056238903, 3.4808797728494074, 3.4808811012331367, 3.480879433958281, 3.4808793142371366, 3.480878669930749, 3.4808793789167716, 3.4808785832577627, 3.4808783140012585, 3.480877944514941, 3.4808782565470624, 3.4808779185845915, 3.4808775062178894, 3.4808768336750346, 3.480877377840251, 3.4808764388454327, 3.4808777526806165, 3.4808765504816748, 3.480877766532824, 3.4808764236460346, 3.4808764661468627, 3.480876139975534, 3.4808756196171355, 3.4808755983940993, 3.480875242392487, 3.480876068778303, 3.480875408450911, 3.4808748825400992, 3.4808748097219686, 3.48087500297719, 3.4808752841218125, 3.480874985372623, 3.4808741408140937]
  out "Waveform Chart ch0":dbl[](graph)=[3.486007276323045, 3.486007488486389, 3.4860073172085833, 3.48600778289756, 3.486007277066716, 3.48600704269229, 3.4860079889516267, 3.4860078053536183, 3.4860074724618775, 3.486007138864972, 3.4860066939855705, 3.4860067073494285, 3.4860081026328706, 3.4860067644334, 3.4860073555280358, 3.486006746645297, 3.4860071738385447, 3.486007186310952, 3.48600725370475, 3.4860066052991687, 3.486006257190876, 3.486006316381739, 3.4860069859057754, 3.486006134020886, 3.486005732796398, 3.486006033273634, 3.486005896848253, 3.4860058348558574, 3.486005886079627, 3.4860058053715766, 3.4860058155929083, 3.486006035777022, 3.4860064007526304, 3.4860053918354876, 3.486004794222689, 3.4860050773537794, 3.4860050350562255, 3.4860057407186464, 3.486005720021455, 3.486005038268717]
  out "Waveform Chart ch3":dbl[](graph)=[3.484656289005541, 3.4846560008441743, 3.484656615282902, 3.484655957764772, 3.4846558086282267, 3.4846558734638053, 3.4846557080367826, 3.484655303529688, 3.484655499138367, 3.484655411504402, 3.4846550658444753, 3.4846550013963715, 3.48465451472455, 3.4846543043778806, 3.48465339269957, 3.4846541844814176, 3.4846533321251676, 3.4846540710961444, 3.4846535638228944, 3.4846522395828106, 3.4846527451616027, 3.484652446319622, 3.4846527202903763, 3.4846518185455593, 3.484652001298707, 3.484652321137677, 3.484651480337147, 3.4846511320023175, 3.4846509773745447, 3.4846505387415254, 3.4846506392876098, 3.4846509382168462, 3.484650517640251, 3.484649642191482, 3.4846509479500116, 3.484650195167144, 3.484650477362746, 3.4846491268155217, 3.48464861471377, 3.4846497184895195]
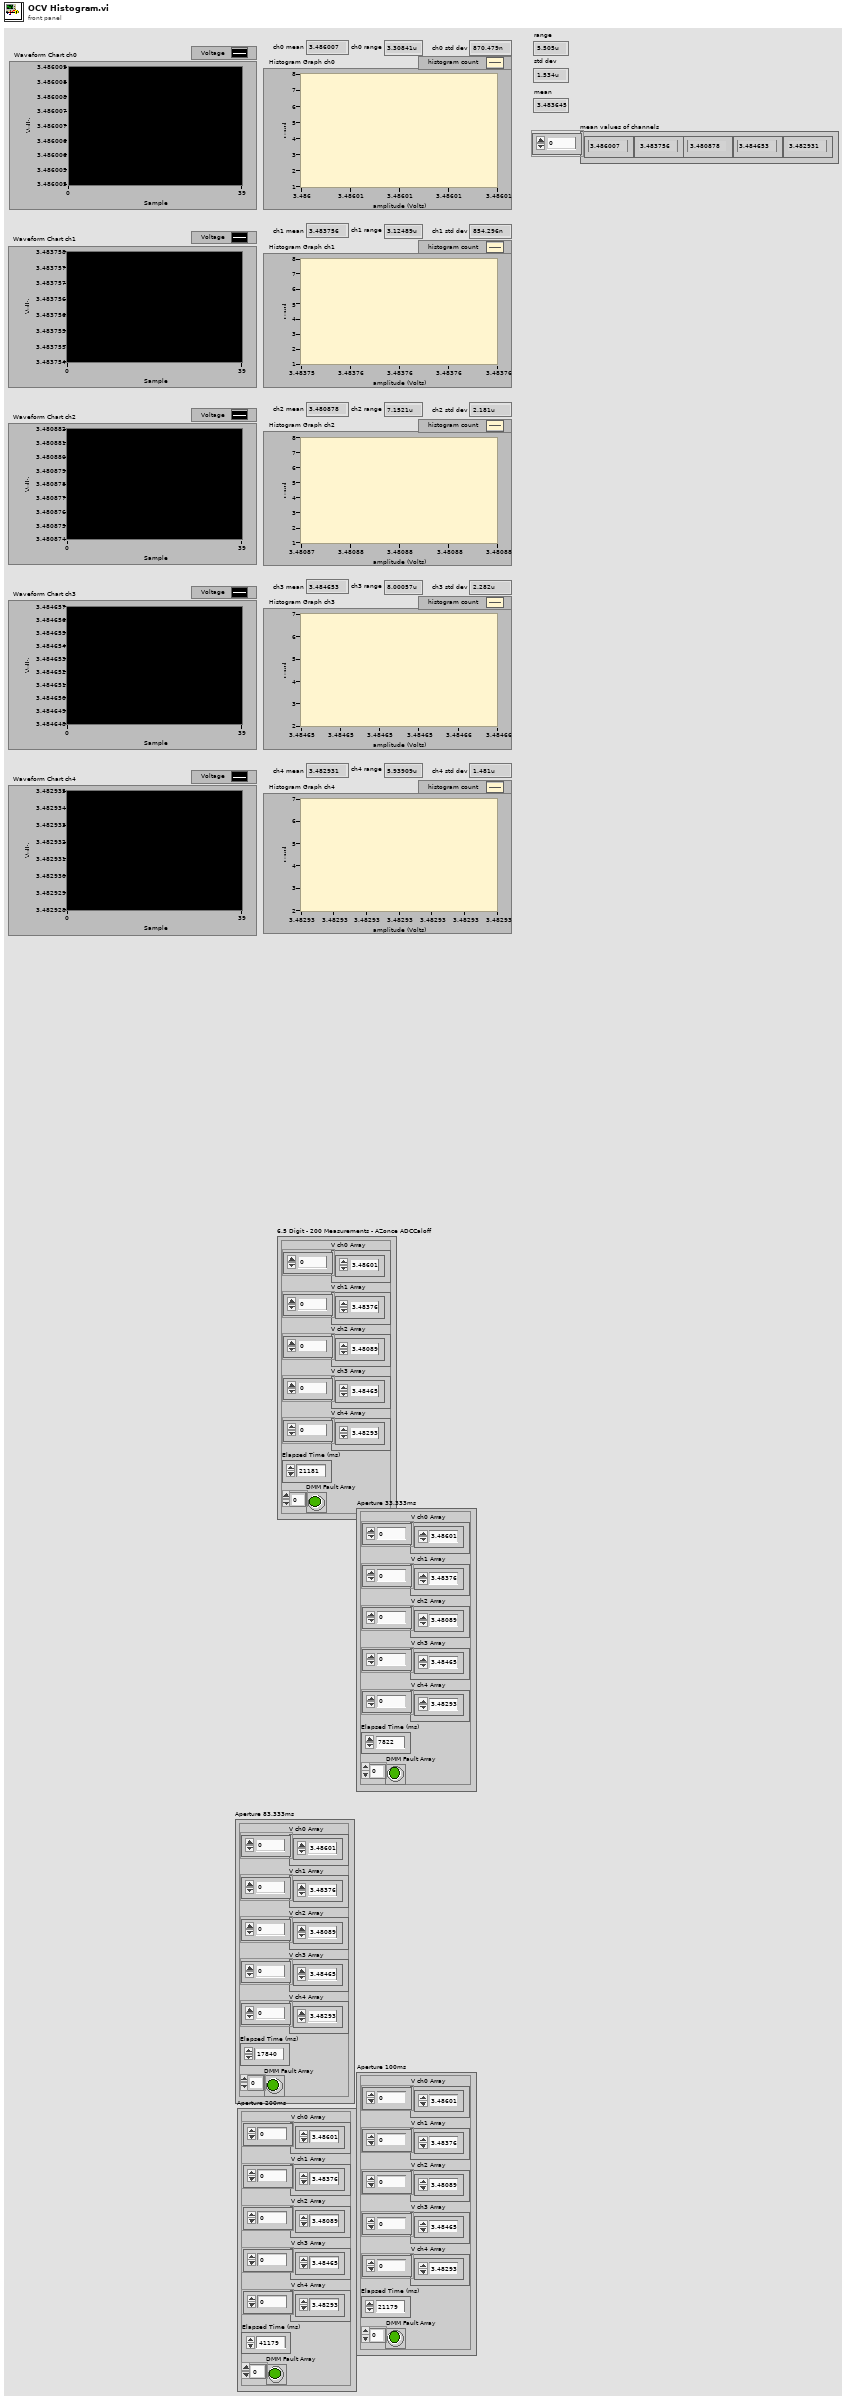
[diagram p1: front panel]
types:
  T1 = typedef "OCVResults.ctl" = cluster{"V ch0 Array":dbl[], "V ch1 Array":dbl[], "V ch2 Array":dbl[], "V ch3 Array":dbl[], "V ch4 Array":dbl[], "Elapsed Time (ms)":u32, "DMM Fault Array":bool[]}
  T2 = cluster{"X Values":dbl[], "Histogram: h(x)":i32[]}
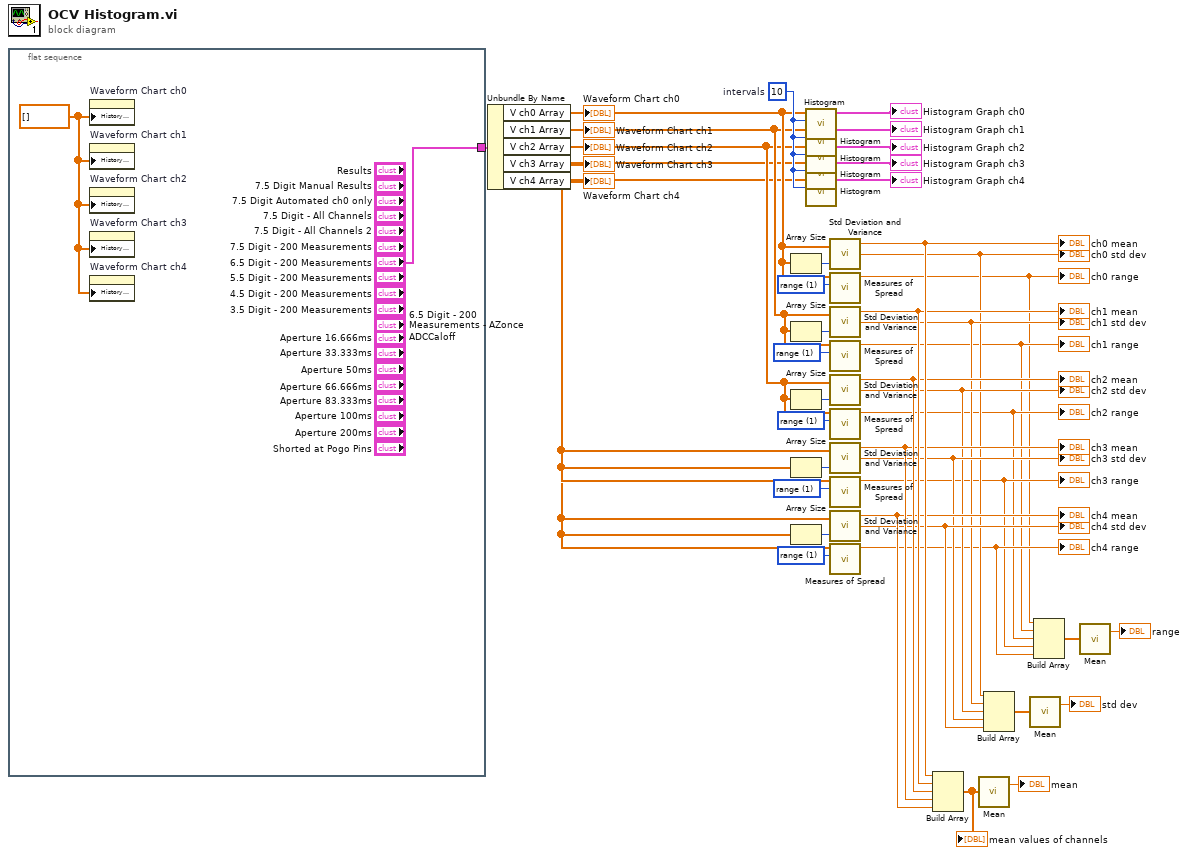
[diagram p0: block diagram]
diagram:
  w24 = 1 items=["standard deviation", "range", "mean absolute deviation", "interquartile range"] ("type")
  w28 = 1 items=["standard deviation", "range", "mean absolute deviation", "interquartile range"] ("type")
  w30 = 1 items=["standard deviation", "range", "mean absolute deviation", "interquartile range"] ("type")
  w33 = 1 items=["standard deviation", "range", "mean absolute deviation", "interquartile range"] ("type")
  w36 = 1 items=["standard deviation", "range", "mean absolute deviation", "interquartile range"] ("type")
  w38 = 10  # intervals
  n1 = flat-sequence {
    tunnel: ["6.5 Digit - 200 Measurements"] -> w1
    frame #0 {
      w45 = dbl[] [] ("History Data")
      n2 = property on="Waveform Chart ch0" class="WFChart (strict)"("History Data"=w45) -> ()  [unwired: 2 in, 2 out]
      n3 = property on="Waveform Chart ch1" class="WFChart (strict)"("History Data"=w45) -> ()  [unwired: 2 in, 2 out]
      n4 = property on="Waveform Chart ch2" class="WFChart (strict)"("History Data"=w45) -> ()  [unwired: 2 in, 2 out]
      n5 = property on="Waveform Chart ch3" class="WFChart (strict)"("History Data"=w45) -> ()  [unwired: 2 in, 2 out]
      n6 = property on="Waveform Chart ch4" class="WFChart (strict)"("History Data"=w45) -> ()  [unwired: 2 in, 2 out]
    }
  }
  n7 = Unbundle By Name(w1) -> ("V ch0 Array"=w35:dbl[], "V ch1 Array"=w32:dbl[], "V ch2 Array"=w27:dbl[], "V ch3 Array"=w26:dbl[], "V ch4 Array"=w23:dbl[])
  "Waveform Chart ch3" <- w26
  "Waveform Chart ch0" <- w35
  "Waveform Chart ch2" <- w27
  "Waveform Chart ch4" <- w23
  "Waveform Chart ch1" <- w32
  n8 = Array Size(array=w35) -> (size(s)=w37:i32)
  n9 = Array Size(array=w32) -> (size(s)=w34:i32)
  n10 = Array Size(array=w27) -> (size(s)=w31:i32)
  n11 = Array Size(array=w26) -> (size(s)=w29:i32)
  n12 = Array Size(array=w23) -> (size(s)=w25:i32)
  n13 = call <vilib>:"Histogram.vi"("intervals"=w38, "X"=w35) -> ("Histogram Graph"=→"Histogram Graph ch0":T2)  [unwired: 6 in, 3 out]
  n14 = call <vilib>:"Histogram.vi"("intervals"=w38, "X"=w32) -> ("Histogram Graph"=→"Histogram Graph ch1":T2)  [unwired: 6 in, 3 out]
  n15 = call <vilib>:"Histogram.vi"("intervals"=w38, "X"=w27) -> ("Histogram Graph"=→"Histogram Graph ch2":T2)  [unwired: 6 in, 3 out]
  n16 = call <vilib>:"Histogram.vi"("intervals"=w38, "X"=w26) -> ("Histogram Graph"=→"Histogram Graph ch3":T2)  [unwired: 6 in, 3 out]
  n17 = call <vilib>:"Histogram.vi"("intervals"=w38, "X"=w23) -> ("Histogram Graph"=→"Histogram Graph ch4":T2)  [unwired: 6 in, 3 out]
  n18 = call <vilib>:"Std Deviation and Variance.vi"("X"=w35, "Weighting (Sample)"=w37) -> ("mean"=w22:dbl, "standard deviation"=w9:dbl)  [unwired: 1 out]
  "ch0 mean" <- w22
  "ch0 std dev" <- w9
  n19 = call <vilib>:"Measures of Spread.vi"("type"=w36, "x array"=w35) -> ("spread value"=w2:dbl)  [unwired: 8 in, 1 out]
  "ch0 range" <- w2
  n20 = call <vilib>:"Std Deviation and Variance.vi"("X"=w32, "Weighting (Sample)"=w34) -> ("mean"=w21:dbl, "standard deviation"=w10:dbl)  [unwired: 1 out]
  "ch1 mean" <- w21
  "ch1 std dev" <- w10
  n21 = call <vilib>:"Measures of Spread.vi"("type"=w33, "x array"=w32) -> ("spread value"=w3:dbl)  [unwired: 8 in, 1 out]
  "ch1 range" <- w3
  n22 = call <vilib>:"Std Deviation and Variance.vi"("X"=w27, "Weighting (Sample)"=w31) -> ("mean"=w20:dbl, "standard deviation"=w11:dbl)  [unwired: 1 out]
  "ch2 mean" <- w20
  "ch2 std dev" <- w11
  n23 = call <vilib>:"Measures of Spread.vi"("type"=w30, "x array"=w27) -> ("spread value"=w4:dbl)  [unwired: 8 in, 1 out]
  "ch2 range" <- w4
  n24 = call <vilib>:"Std Deviation and Variance.vi"("X"=w26, "Weighting (Sample)"=w29) -> ("mean"=w19:dbl, "standard deviation"=w12:dbl)  [unwired: 1 out]
  "ch3 mean" <- w19
  "ch3 std dev" <- w12
  n25 = call <vilib>:"Measures of Spread.vi"("type"=w28, "x array"=w26) -> ("spread value"=w5:dbl)  [unwired: 8 in, 1 out]
  "ch3 range" <- w5
  n26 = call <vilib>:"Std Deviation and Variance.vi"("X"=w23, "Weighting (Sample)"=w25) -> ("mean"=w18:dbl, "standard deviation"=w13:dbl)  [unwired: 1 out]
  "ch4 mean" <- w18
  "ch4 std dev" <- w13
  n27 = call <vilib>:"Measures of Spread.vi"("type"=w24, "x array"=w23) -> ("spread value"=w6:dbl)  [unwired: 8 in, 1 out]
  "ch4 range" <- w6
  n28 = Build Array(w22, w21, w20, w19, w18) -> (w17:dbl[])
  "mean values of channels" <- w17
  n29 = call-poly <vilib>:"Mean.vi"("X"=w17) -> ("mean"=→"mean":dbl)  [unwired: 1 out]
  n30 = Build Array(w9, w10, w11, w12, w13) -> (w15:dbl[])
  n31 = call-poly <vilib>:"Mean.vi"("X"=w15) -> ("mean"=→"std dev":dbl)  [unwired: 1 out]
  n32 = Build Array(w2, w3, w4, w5, w6) -> (w8:dbl[])
  n33 = call-poly <vilib>:"Mean.vi"("X"=w8) -> ("mean"=→"range":dbl)  [unwired: 1 out]
